vi "CRYGraph XY Window.vi"() -> ()   [LabVIEW 2013]
uses:
  <vilib>/Utility/miscctls.llb/LVPoint32TypeDef.ctl
  Control/CRYFlag Cluster.ctl
  <vilib>/Utility/miscctls.llb/LVRowAndColumnTypeDef.ctl
  <vilib>/Utility/miscctls.llb/LVRectTypeDef.ctl
  CRYCurveLibrary/Global/CRYCurve Library Global.vi
  SubVI/CRYData View Global.vi
  SubVI/CRYMain Sub Window Global.vi
panel:
  in  "GraphClick":bool
  out "AxisChangeOption":string
  out "PhaseShow":bool=TRUE
  in  "WhichKey":string
  out "KeyRepeatCount":i32
  in  "CursorMoveFinish":bool
  out "LegendVScrollShow":bool=TRUE
  out "Legend Ref":refnum<vi>
  out "SelectedRow":i32[](array[numeric])
  in  "LoadFinish":bool
  in  "ScaleFitY 2":bool
  in  "ScaleFitY":bool
  in  "ScaleFitX":bool
  in  "ToolbarUpdate":bool
  in  "OpenProperty":bool
  out "PropertyTab":string
  in  "PaletteShow":bool
  out "PreviewScaleMin":dbl
  out "PreviewScaleMax":dbl
  in  "FitPanes":bool
  in  "DirectionKey":bool
  out "MagnitudeShow":bool=TRUE
  out "Graph Ref":refnum<vi>
  out "PreviewGraph Ref":refnum<vi>
  out "PreviewCoords":T1
  in  "ScaleRange":bool
  out "Repaint Watermark":i32
  out "Event Name":string
  out "ReportDrop":bool
  in  "AxisChange":bool
  in  "RemoveSome":bool
  out "ScaleMin":dbl
  out "ScaleMax":dbl
  out "ScrollTick Ref":refnum<vi>
  out "Scrollbar Ref":refnum<vi>
  in  "PreviewShow":bool
  in  "RemoveAll":bool
  in  "CursorColor":bool
  out "NewCursIdx":u32
  out "Test":string
  in  "OldCursIdx":u32
  out "Queue Name":string
  in  "StateOut":bool
  out "Cursor Coords":T1
  in  "CursorPlot":bool
  out "Cursor Ref":refnum<vi>
  in  "CursorShow":bool
  out "XY Graph":cluster{"XY Graph":cluster{dbl, dbl}[]}[](graph)
  out "Title Name":string
  out "OldRow":i32
  out "TotalPlot":u32
  out "Graph Number":i32
  in  "stop":bool
  out "PreviewGraph":cluster{"XY Graph":cluster{dbl, dbl}[]}[](graph)
  in  "CursorEnabled":bool
  in  "Scrollbar":dbl(c297)
  in  "ScrollTick":dbl(slide) scale=0.0..1.0 scale format="%-#3.2p"
  in  "Cursor":string[][](table)
  in  "LegendShow":bool
  in  "ColorBox":u32(colorbox)
  in  "Legend":i32[](listbox)
  in  "GraphType":string
types:
  T1 = typedef "LVPoint32TypeDef.ctl" = cluster{"Horizontal":i32, "Vertical":i32}
  T2 = typedef "CRYFlag Cluster.ctl" = cluster{"LegendShow":bool, "CellClick":bool, "Total Number":bool, "ScaleFitX":bool, "ScaleFitY":bool, "MapModeX":u8, "MapModeY":u8, "CursorShow":bool, "MagnitudeShow":bool, "PreviewShow":bool, "CursorEnabled":bool, "IntensityShow":bool, "PaletteShow":bool, "PhaseShow":bool, "XYShow":bool, "FrequencyShow":bool, "LegendVScrollShow":bool, "FrequencyVScrollShow":bool}
  T3 = typedef "CRYGraph Event.ctl" = cluster{"EvenName":string, "TitleName":string, "GraphName":string, "GraphType":string, "Data":variant, "Queue Name":string, "DataView Number":i32}
  T4 = enum16{"No Scaling", "Scale All Objects", "Scale Single Object"}
  T5 = typedef "LVRowAndColumnTypeDef.ctl" = cluster{"Row":i32, "Column":i32}
  T6 = typedef "LVRectTypeDef.ctl" = cluster{"Left":i16, "Top":i16, "Right":i16, "Bottom":i16}
  T7 = typedef "LVBoundsTypeDef.ctl" = cluster{"Width":u32, "Height":u32}
  T8 = typedef "LVPositionTypeDef.ctl" = cluster{"Left":i32, "Top":i32}
  T9 = typedef "CRYData Cluster.ctl" = cluster{"Name":string, "Curve":cluster{"x":dbl, "y":dbl, "z":dbl}[], "X data":u16, "Y data":u16, "Z data":u16, "X axis":u16, "Y axis":u16, "Z axis":u16, "X unit":string, "Y unit":string, "Z unit":string, "X dB ref":dbl, "Y dB ref":dbl, "Z dB ref":dbl, "single val":bool, "protected":bool, "display X":bool, "display Y":bool, "display Z":bool, "Test Info":string, "Step No.":i32, "Plot Settings":cluster{"Color":u32, "Interpolation":u8, "Point Style":u8, "Line Style":u8, "Point Color":u32, "Line Width":u8, "Bar Plot Style":u8, "Fill To":i16}, "AutoProtect":bool}
  T10 = typedef "LVRangeTypeDef.ctl" = cluster{"Minimum":dbl, "Maximum":dbl, "Increment":dbl, "Minor Increment":dbl, "Start":dbl}
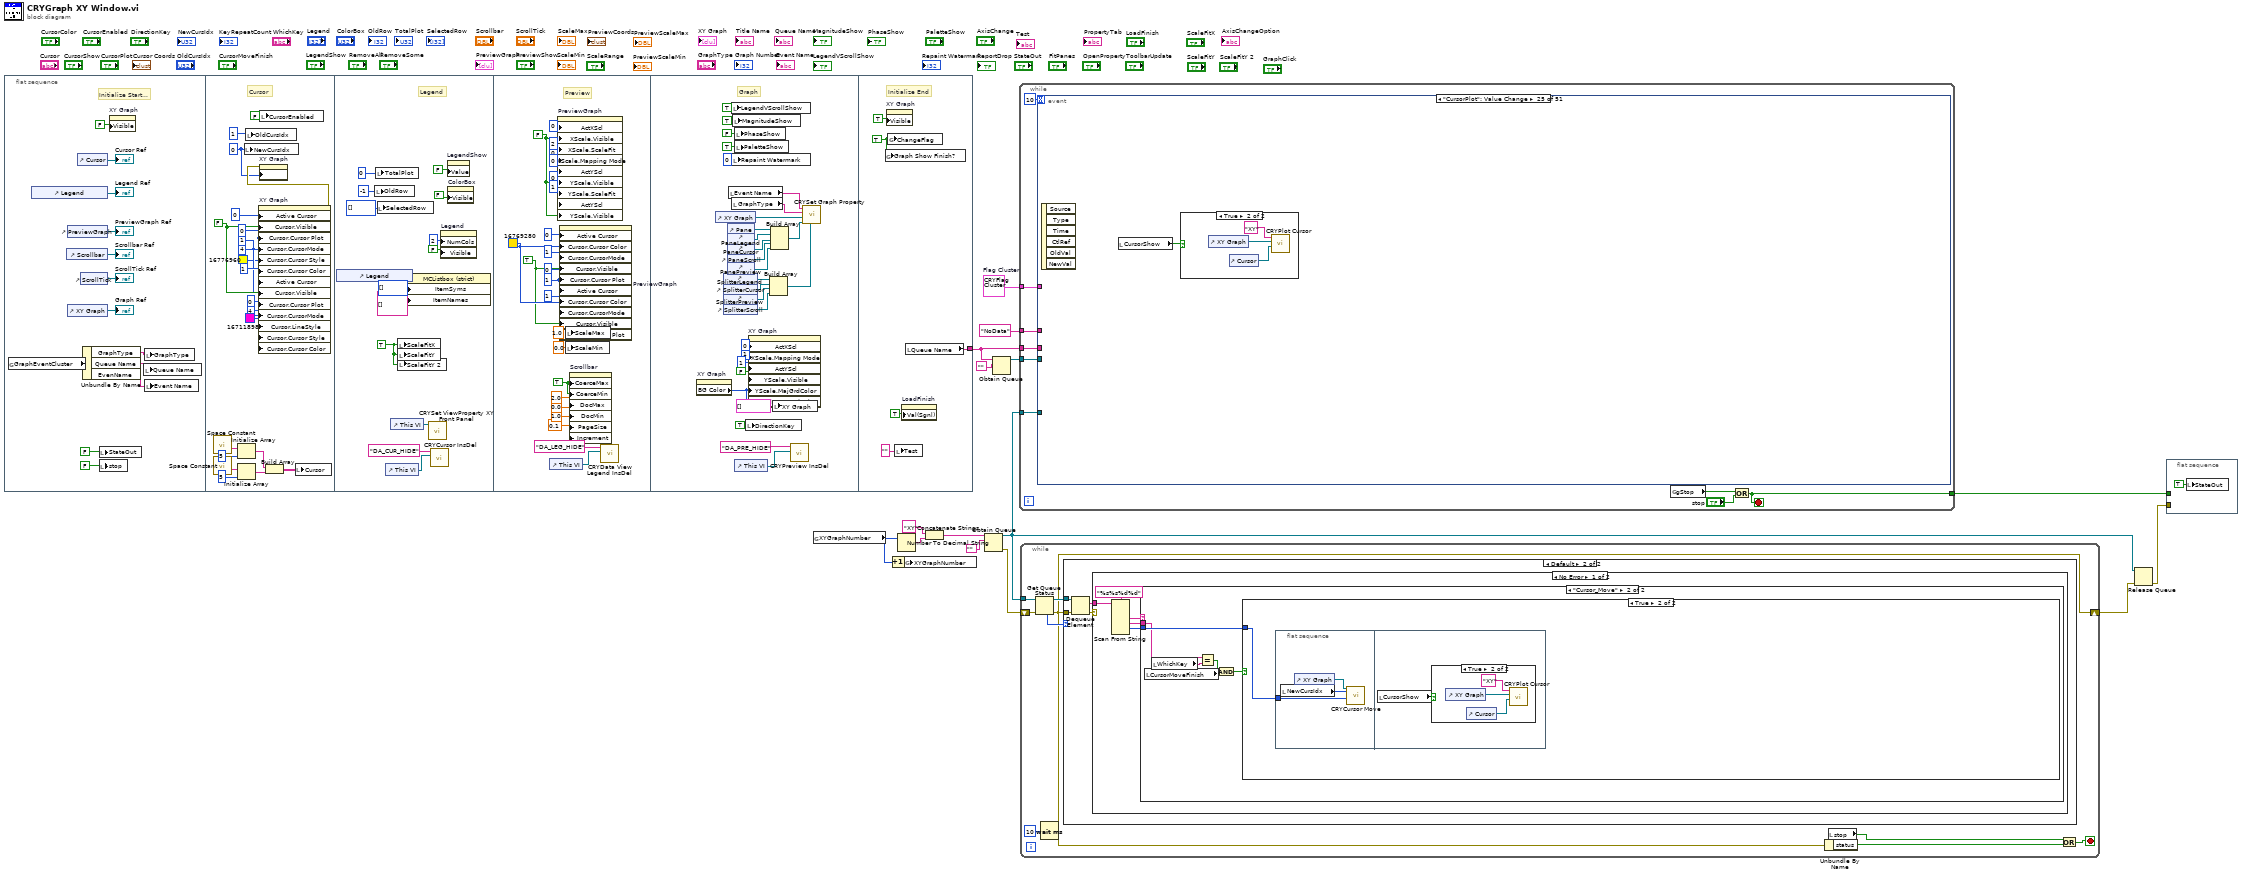
[diagram p0: block diagram]
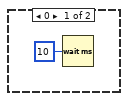
[diagram p2: hidden frame]
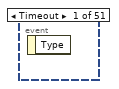
[diagram p7: hidden frame]
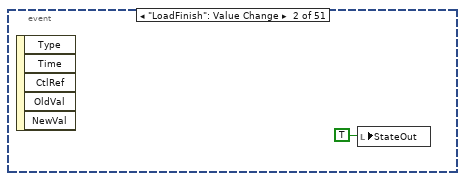
[diagram p8: hidden frame]
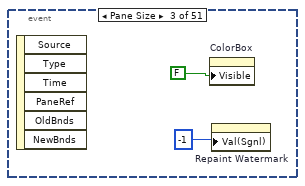
[diagram p9: hidden frame]
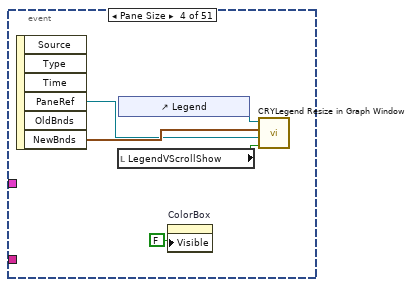
[diagram p10: hidden frame]
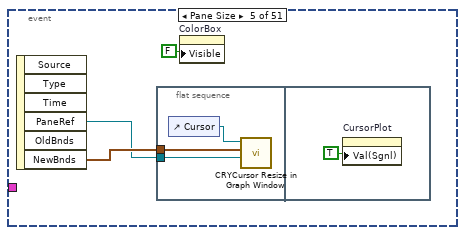
[diagram p11: hidden frame]
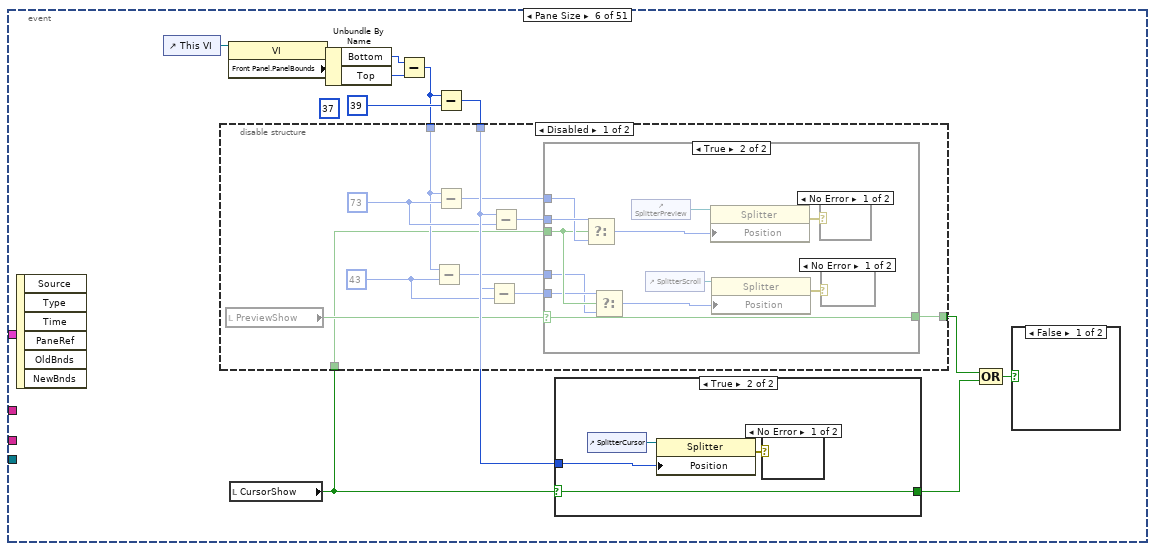
[diagram p12: hidden frame]
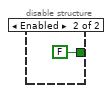
[diagram p16: hidden frame]
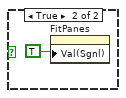
[diagram p17: hidden frame]
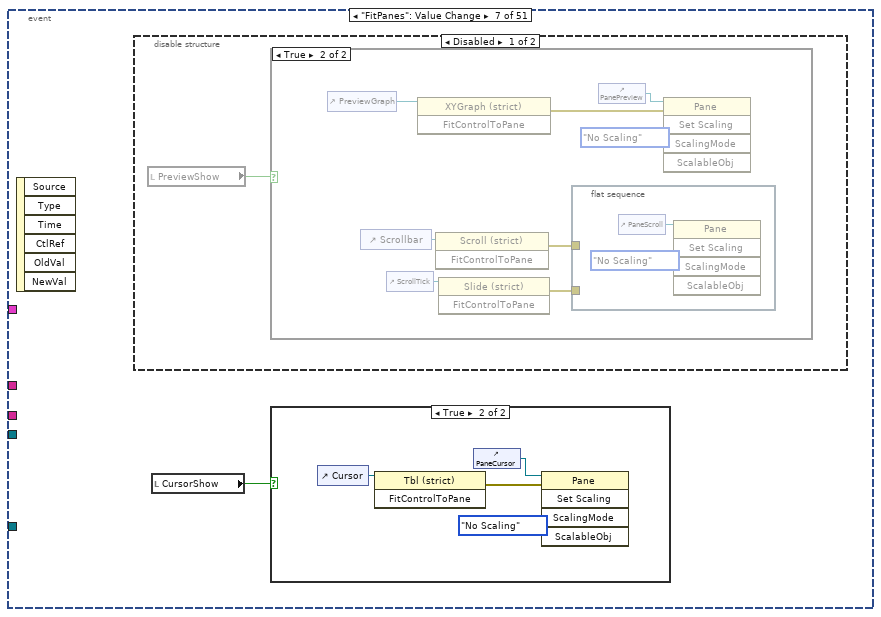
[diagram p20: hidden frame]
diagram:
  w14 = T2 {"LegendShow"=FALSE, "CellClick"=FALSE, "Total Number"=FALSE, "ScaleFitX"=FALSE, "ScaleFitY"=FALSE, "MapModeX"=0, "MapModeY"=0, "CursorShow"=FALSE, "MagnitudeShow"=FALSE, "PreviewShow"=FALSE, "CursorEnabled"=FALSE, "IntensityShow"=FALSE, "PaletteShow"=FALSE, "PhaseShow"=FALSE, "XYShow"=FALSE, "FrequencyShow"=FALSE, "LegendVScrollShow"=FALSE, "FrequencyVScrollShow"=FALSE}  # Flag Cluster
  n1 = flat-sequence {
    tunnel: [w117] -> w12
    frame #0 {
      # "Initialize Start..."
      n2 = global read "CRYData View Global.vi" "GraphEventCluster"() -> (w23:T3)
      n3 = control-ref of="Legend"() -> (→"Legend Ref":refnum<vi>)
      n4 = control-ref of="Scrollbar"() -> (→"Scrollbar Ref":refnum<vi>)
      n5 = control-ref of="PreviewGraph"() -> (→"PreviewGraph Ref":refnum<vi>)
      n6 = control-ref of="XY Graph"() -> (→"Graph Ref":refnum<vi>)
      n7 = control-ref of="Cursor"() -> (→"Cursor Ref":refnum<vi>)
      n8 = control-ref of="ScrollTick"() -> (→"ScrollTick Ref":refnum<vi>)
      n9 = Unbundle By Name(w23) -> ("GraphType"=w21:string, "Queue Name"=w22:string, "EvenName"=w20:string)
      n10 = local write "StateOut"(FALSE ("StateOut")) -> ()
      n11 = local write "stop"(FALSE ("stop")) -> ()
      n12 = property on="XY Graph" class="XYGraph (strict)"("Visible"=FALSE) -> ()  [unwired: 2 in, 2 out]
      n13 = local write "Queue Name"(w22) -> ()
      n14 = local write "GraphType"(w21) -> ()
      n15 = local write "Event Name"(w20) -> ()
    }
    frame #1 {
      w34 = u32 0 ("Active Cursor")
      w36 = u32 1 ("Cursor.Cursor Mode")
      w37 = 0 ("Cursor.Cursor Plot")
      w38 = FALSE ("Cursor.Visible")
      # "Cursor"
      n16 = call <vilib>:"Space Constant.vi"() -> ("String"=w44:string)
      n17 = call <vilib>:"Space Constant.vi"() -> ("String"=w49:string)
      n18 = Initialize Array(w44, 5 ("dimension size")) -> (w46:string[])
      n19 = Initialize Array(w49, 5 ("dimension size")) -> (w50:string[])
      n20 = local write "NewCursIdx"(w34) -> ()
      n21 = local write "OldCursIdx"(u32 1 ("OldCursIdx")) -> ()
      n22 = property on="XY Graph" class="XYGraph (strict)"("Active Cursor"=u32 0, "Cursor.Visible"=w38, "Cursor.Cursor Plot"=w37, "Cursor.CursorMode"=w36, "Cursor.Cursor Style"=u8 4, "Cursor.Cursor Color"=u32 16776960, "Active Cursor"=u32 1, "Cursor.Visible"=w38, "Cursor.Cursor Plot"=w37, "Cursor.CursorMode"=w36, "Cursor.LineStyle"=u8 0 ("Cursor.Line Style"), "Cursor.Cursor Style"=u8 4, "Cursor.Cursor Color"=u32 16711898) -> (error out=w35:errorcluster)  [unwired: 2 in, 1 out]
      n23 = property on="XY Graph" class="XYGraph (strict)"(error in=w35, "Active Cursor"=w34) -> ()  [unwired: 1 in, 2 out]
      n24 = local write "CursorEnabled"(FALSE ("CursorEnabled")) -> ()
      n25 = Build Array(w46, w50) -> (w47:string[][])
      n26 = local write "Cursor"(w47) -> ()
    }
    frame #2 {
      w52 = TRUE ("ScaleFitX")
      # "Legend"
      n27 = control-ref of="Legend"() -> (w64:refnum<vi>)
      n28 = local write "OldRow"(-1 ("OldRow 2")) -> ()
      n29 = local write "TotalPlot"(u32 0 ("TotalPlot")) -> ()
      n30 = local write "SelectedRow"(i32[] [] ("SelectedRow")) -> ()
      n31 = control-ref of="This VI"() -> (w55:refnum<vi>)
      n32 = control-ref of="This VI"() -> (w53:refnum<vi>)
      n33 = local write "ScaleFitX"(w52) -> ()
      n34 = local write "ScaleFitY"(w52) -> ()
      n35 = local write "ScaleFitY 2"(w52) -> ()
      n36 = property on="Property Node" class="MCListbox (strict)"(reference=w64, "ItemSyms"=i32[] [] ("Item Symbols"), "ItemNames"=string[][] [] ("Item Names")) -> ()  [unwired: 1 in, 2 out]
      n37 = call "CRYSet ViewProperty XY  Front Panel.vi"("Vi Ref"=w53) -> ()  [unwired: 11 in]
      n38 = call "CRYCursor InsDel.vi"("Graph VI Ref"=w55, "sAction"="DA_CUR_HIDE" ("Action Type")) -> ()  [unwired: 10 in]
      n39 = property on="Legend" class="MCListbox (strict)"("NumCols"=u32 2 ("Number of Columns"), "Visible"=FALSE) -> ()  [unwired: 2 in, 2 out]
      n40 = property on="LegendShow" class="Bool (strict)"("Value"=FALSE ("Visible")) -> ()  [unwired: 2 in, 2 out]
      n41 = property on="ColorBox" class="ColBox"("Visible"=FALSE) -> ()  [unwired: 2 in, 2 out]
    }
    frame #3 {
      w72 = 0 ("Cursor.Cursor Plot")
      w68 = u32 16769280
      w67 = TRUE ("Cursor.Visible")
      w65 = FALSE ("X Scale.Visible")
      w87 = TRUE ("Coerce Maximum Value")
      # "Preview"
      n42 = control-ref of="This VI"() -> (w75:refnum<vi>)
      n43 = property on="PreviewGraph" class="XYGraph (strict)"("ActXScl"=0 ("Active X Scale"), "XScale.Visible"=w65, "XScale.ScaleFit"=u8 2 ("X Scale.Scale Fit"), "XScale.Mapping Mode"=u8 0 ("X Scale.Mapping Mode"), "ActYScl"=0 ("Active Y Scale"), "YScale.Visible"=w65, "YScale.ScaleFit"=u8 0 ("Y Scale.Scale Fit"), "ActYScl"=1 ("Active Y Scale"), "YScale.Visible"=w65) -> ()  [unwired: 2 in, 2 out]
      n44 = property on="PreviewGraph" class="XYGraph (strict)"("Active Cursor"=u32 0, "Cursor.Cursor Color"=w68, "Cursor.CursorMode"=u32 1 ("Cursor.Cursor Mode"), "Cursor.Visible"=w67, "Cursor.Cursor Plot"=w72, "Active Cursor"=u32 1, "Cursor.Cursor Color"=w68, "Cursor.CursorMode"=u32 1 ("Cursor.Cursor Mode"), "Cursor.Visible"=w67, "Cursor.Cursor Plot"=w72) -> ()  [unwired: 2 in, 2 out]
      n45 = local write "ScaleMax"(1.0 ("ScaleMax")) -> ()
      n46 = local write "ScaleMin"(0.0 ("ScaleMin")) -> ()
      n47 = property on="Scrollbar" class="Scroll (strict)"("CoerceMax"=w87, "CoerceMin"=w87, "DocMax"=2.0 ("Doc Max"), "DocMin"=0.0 ("Doc Min"), "PageSize"=1.0 ("Page Size"), "Increment"=0.1) -> ()  [unwired: 2 in, 2 out]
      n48 = call "CRYData View Legend InsDel.vi"("Graph VI Ref"=w75, "sAction"="DA_LEG_HIDE" ("Action Type")) -> ()  [unwired: 2 in, 8 out]
    }
    frame #4 {
      # "Graph"
      n49 = property on="XY Graph" class="XYGraph (strict)"() -> ("BG Color"=w113:u32)  [unwired: 2 in, 2 out]
      n50 = control-ref of="XY Graph"() -> (w96:refnum<vi>)
      n51 = control-ref of="SplitterLegend"() -> (w110:refnum<vi>)
      n52 = control-ref of="SplitterCursor"() -> (w109:refnum<vi>)
      n53 = control-ref of="SplitterPreview"() -> (w108:refnum<vi>)
      n54 = control-ref of="SplitterScroll"() -> (w107:refnum<vi>)
      n55 = control-ref of="Pane"() -> (w106:refnum<vi>)
      n56 = control-ref of="PaneLegend"() -> (w102:refnum<vi>)
      n57 = control-ref of="PaneCursor"() -> (w105:refnum<vi>)
      n58 = control-ref of="PaneScroll"() -> (w104:refnum<vi>)
      n59 = control-ref of="PanePreview"() -> (w103:refnum<vi>)
      n60 = local read "Event Name"() -> (w98:string)
      n61 = local write "LegendVScrollShow"(TRUE ("LegendVScrollShow")) -> ()
      n62 = local write "Repaint Watermark"(0 ("Repaint Watermark")) -> ()
      n63 = local read "GraphType"() -> (w99:string)
      n64 = local write "MagnitudeShow"(TRUE ("Magnitude")) -> ()
      n65 = local write "PhaseShow"(FALSE ("PhaseShow")) -> ()
      n66 = local write "PaletteShow"(TRUE ("PaletteShow")) -> ()
      n67 = control-ref of="This VI"() -> (w111:refnum<vi>)
      n68 = local write "DirectionKey"(TRUE ("DirectionKey")) -> ()
      n69 = property on="XY Graph" class="XYGraph (strict)"("ActXScl"=0 ("Active X Scale"), "XScale.Mapping Mode"=u8 1 ("X Scale.Mapping Mode"), "ActYScl"=1 ("Active Y Scale"), "YScale.Visible"=FALSE ("Y Scale.Visible"), "YScale.MajGrdColor"=w113, "YScale.MnrGrdColor"=w113) -> ()  [unwired: 2 in, 2 out]
      n70 = Build Array(w110, w109, w108, w107) -> (w100:refnum<vi>[])
      n71 = Build Array(w106, w102, w105, w104, w103) -> (w101:refnum<vi>[])
      n72 = local write "XY Graph"(cluster{"XY Graph":cluster{dbl, dbl}[]}[] [] ("XY Graph")) -> ()
      n73 = call "CRYPreview InsDel.vi"("Graph VI Ref"=w111, "sAction"="DA_PRE_HIDE" ("Action Type")) -> ()  [unwired: 10 in]
      n74 = call "CRYSet Graph Property.vi"("Splitters"=w100, "Panes"=w101, "Graph Ref"=w96, "Graph Type"=w99, "Event Name"=w98) -> ()  [unwired: 7 in]
    }
    frame #5 {
      w120 = TRUE ("ChangeFlag")
      # "Initialize End"
      n75 = global write "CRYData View Global.vi" "Graph Show Finish?"(w120) -> ()
      n76 = property on="XY Graph" class="XYGraph (strict)"("Visible"=TRUE) -> ()  [unwired: 2 in, 2 out]
      n77 = global write "CRYData View Global.vi" "ChangeFlag"(w120) -> ()
      n78 = local write "Test"("" ("Test")) -> ()
      n79 = property on="LoadFinish" class="Bool (strict)"("Val(Sgnl)"=TRUE ("Value (Signaling)")) -> ()  [unwired: 2 in, 2 out]
      n80 = local read "Queue Name"() -> (w117:string)
    }
  }
  n81 = global read "CRYCurve Library Global.vi" "XYGraphNumber"() -> (w4:u32)
  n82 = Increment(x=w4) -> (x+1=w3:u32)
  n83 = Number To Decimal String(number=w4) -> (decimal integer string=w5:string)  [unwired: 1 in]
  n84 = global write "CRYCurve Library Global.vi" "XYGraphNumber"(w3) -> ()
  n85 = Concatenate Strings("XY" ("YAxisTitle"), w5) -> (w7:string)
  n86 = Obtain Queue(name (unnamed)=w7, element data type="" ("Action Type")) -> (queue out=w1:refnum<queue>, error out=w10:errorcluster)  [unwired: 3 in, 1 out]
  n87 = Obtain Queue(name (unnamed)=w12, element data type="") -> (queue out=w16:refnum<queue>)  [unwired: 3 in, 2 out]
  n88 = while {
    tunnel: w16 -> [w129]
    tunnel: w14 -> [w127]
    tunnel: "NoData" ("input 2") -> [w124]
    tunnel: w12 -> [w123]
    tunnel: [w122] -> w11
    tunnel: w1 -> [w121]
    stop <- w122 stop-if-true
    n89 = event shown="[24] \"CursorPlot\": Value Change" {
      selector: _ -> [_ _ _ _ _ _ _ _ _ _ _ _ _ _ _ _ _ _ _ _ _ _ _ _ _ _ _ _ _ _ _ _ _ _ _ _ _ _ _ _ _ _ _ _ _ _ _ _ _ _ _]
      dyn-events: _ -> [_ _ _ _ _ _ _ _ _ _ _ _ _ _ _ _ _ _ _ _ _ _ _ _ _ _ _ _ _ _ _ _ _ _ _ _ _ _ _ _ _ _ _ _ _ _ _ _ _ _ _]
      timeout: 10 -> [_ _ _ _ _ _ _ _ _ _ _ _ _ _ _ _ _ _ _ _ _ _ _ _ _ _ _ _ _ _ _ _ _ _ _ _ _ _ _ _ _ _ _ _ _ _ _ _ _ _ _]
      tunnel: w129 -> [_ _ _ _ _ _ _ w205 w210 _ w246 _ w454 _ w507 _ _ _ _ _ _ _ _ _ _ _ _ _ _ _ _ w810 _ _ _ _ _ w1065 _ _ w1078 _ _ _ _ _ _ _ _ _ _]
      tunnel: w127 -> [_ _ _ _ _ _ _ _ _ w230 _ w431 _ w492 _ w550 _ _ _ _ _ _ _ _ _ _ _ _ _ _ _ _ _ _ _ _ _ _ _ _ _ _ _ _ _ _ _ _ _ _ _]
      tunnel: w124 -> [_ _ _ _ _ _ _ _ _ _ w248 _ w451 _ w506 _ _ _ _ _ _ _ _ _ _ _ _ _ _ _ _ _ _ _ _ _ _ _ _ _ _ _ _ _ _ _ _ _ _ _ _]
      tunnel: w123 -> [_ _ _ _ _ _ _ _ _ w223 w247 _ _ _ _ _ _ _ _ _ _ _ _ _ _ _ _ _ _ _ _ _ _ _ _ _ _ _ _ _ _ _ _ _ _ _ _ _ _ _ _]
      tunnel: w121 -> [_ _ _ _ _ _ _ _ _ _ _ _ _ _ _ _ _ _ w634 w653 w668 _ _ _ _ _ _ _ _ _ _ _ _ _ _ _ _ _ _ _ _ _ _ _ _ _ _ _ _ _ _]
      event Timeout {
        n90 = event-data() -> ()  [unwired: 2 out]
      }
      event "LoadFinish": Value Change {
        n91 = event-data() -> ()  [unwired: 6 out]
        n92 = local write "StateOut"(TRUE ("StateOut")) -> ()
      }
      event Pane Size {
        n93 = event-data() -> ()  [unwired: 7 out]
        n94 = property on="ColorBox" class="ColBox"("Visible"=FALSE) -> ()  [unwired: 2 in, 2 out]
        n95 = property on="Repaint Watermark" class="DigNum (strict)"("Val(Sgnl)"=-1 ("y")) -> ()  [unwired: 2 in, 2 out]
      }
      event Pane Size {
        n96 = event-data() -> ("PaneRef"=w135:refnum<vi>, "NewBnds"=w136:T6)  [unwired: 5 out]
        n97 = local read "LegendVScrollShow"() -> (w133:bool)
        n98 = control-ref of="Legend"() -> (w134:refnum<vi>)
        n99 = property on="ColorBox" class="ColBox"("Visible"=FALSE) -> ()  [unwired: 2 in, 2 out]
        n100 = call "CRYLegend Resize in Graph Window.vi"("VScrollShow"=w133, "Pane Ref"=w135, "input cluster"=w136, "Legend"=w134) -> ()  [unwired: 8 out]
      }
      event Pane Size {
        n101 = event-data() -> ("PaneRef"=w139:refnum<vi>, "NewBnds"=w140:T6)  [unwired: 5 out]
        n102 = flat-sequence {
          tunnel: w140 -> [w143]
          tunnel: w139 -> [w141]
          frame #0 {
            n103 = control-ref of="Cursor"() -> (w142:refnum<vi>)
            n104 = call "CRYCursor Resize in Graph Window.vi"("Pane Ref"=w141, "input cluster"=w143, "Graph Cursor Ref"=w142) -> ()  [unwired: 9 in]
          }
          frame #1 {
            n105 = property on="CursorPlot" class="Bool (strict)"("Val(Sgnl)"=TRUE ("Value (Signaling)")) -> ()  [unwired: 2 in, 2 out]
          }
        }
        n106 = property on="ColorBox" class="ColBox"("Visible"=FALSE) -> ()  [unwired: 2 in, 2 out]
      }
      event Pane Size {
        (unwired) 37
        n107 = event-data() -> ()  [unwired: 7 out]
        n108 = control-ref of="This VI"() -> (w149:refnum<vi>)
        n109 = property class="VI"(reference=w149) -> ("Front Panel.PanelBounds"=w150:T6)  [unwired: 1 in, 2 out]
        n110 = local read "CursorShow"() -> (w146:bool)
        n111 = Unbundle By Name(w150) -> ("Bottom"=w147:i16, "Top"=w148:i16)
        n112 = Subtract(x=w147, y=w148) -> (x-y=w151:i16)
        n113 = Subtract(x=w151, y=39) -> (x-y=w155:i32)
        n114 = disable-structure shown="Disabled" {
          disable-tunnel: w155 -> [w163 _]
          disable-tunnel: [w161 FALSE] -> w152
          disable-tunnel: w151 -> [w158 _]
          disable-tunnel: w146 -> [w156 _]
          frame Disabled {
            w164 = 43
            w162 = 73
            n115 = local read "PreviewShow"() -> (w157:bool)
            n116 = Subtract(x=w158, y=w164) -> (x-y=w160:i32)
            n117 = Subtract(x=w158, y=w162) -> (x-y=w159:i32)
            n118 = Subtract(x=w163, y=w164) -> (x-y=w166:i32)
            n119 = Subtract(x=w163, y=w162) -> (x-y=w165:i32)
            n120 = case shown="True" w157 {
              selector: w157 -> [w167 w177]
              tunnel: w159 -> [_ w175]
              tunnel: w160 -> [_ w171]
              tunnel: [w167 w177] -> w161
              tunnel: w156 -> [_ w173]
              tunnel: w165 -> [_ w176]
              tunnel: w166 -> [_ w172]
              frame False {
              }
              frame True {
                n121 = Select(t=w176, s=w173, f=w175) -> (s? t:f=w174:i32)
                n122 = Select(t=w172, s=w173, f=w171) -> (s? t:f=w170:i32)
                n123 = control-ref of="SplitterPreview"() -> (w169:refnum<vi>)
                n124 = control-ref of="SplitterScroll"() -> (w168:refnum<vi>)
                n125 = property class="Splitter"(reference=w169, "Position"=w174) -> (error out=w179:errorcluster)  [unwired: 1 in, 1 out]
                n126 = property class="Splitter"(reference=w168, "Position"=w170) -> (error out=w178:errorcluster)  [unwired: 1 in, 1 out]
                n127 = case shown="No Error" w179 {
                  frame No Error {
                  }
                  frame Error {
                  }
                }
                n128 = case shown="No Error" w178 {
                  frame No Error {
                  }
                  frame Error {
                  }
                }
              }
            }
          }
          frame Enabled {
          }
        }
        n129 = case shown="True" w146 {
          selector: w146 -> [w182 w184]
          tunnel: w155 -> [_ w186]
          tunnel: [w182 w184] -> w153
          frame False {
          }
          frame True {
            n130 = control-ref of="SplitterCursor"() -> (w183:refnum<vi>)
            n131 = property class="Splitter"(reference=w183, "Position"=w186) -> (error out=w185:errorcluster)  [unwired: 1 in, 1 out]
            n132 = case shown="No Error" w185 {
              frame No Error {
              }
              frame Error {
              }
            }
          }
        }
        n133 = Compound Arithmetic op=OR(w152, w153) -> (w145:bool)
        n134 = case shown="False" w145 {
          frame False {
          }
          frame True {
            n135 = property on="FitPanes" class="Bool (strict)"("Val(Sgnl)"=TRUE ("Value (Signaling)")) -> ()  [unwired: 2 in, 2 out]
          }
        }
      }
      event "FitPanes": Value Change {
        n136 = event-data() -> ()  [unwired: 7 out]
        n137 = disable-structure shown="Disabled" {
          frame Disabled {
            n138 = local read "PreviewShow"() -> (w188:bool)
            n139 = case shown="True" w188 {
              frame False {
              }
              frame True {
                n140 = control-ref of="PreviewGraph"() -> (w195:refnum<vi>)
                n141 = control-ref of="Scrollbar"() -> (w194:refnum<vi>)
                n142 = control-ref of="ScrollTick"() -> (w193:refnum<vi>)
                n143 = invoke class="XYGraph (strict)" method="FitControlToPane"(reference=w195) -> (error out=w192:errorcluster)  [unwired: 2 in, 2 out]
                n144 = invoke class="Scroll (strict)" method="FitControlToPane"(reference=w194) -> (error out=w191:errorcluster)  [unwired: 2 in, 2 out]
                n145 = invoke class="Slide (strict)" method="FitControlToPane"(reference=w193) -> (error out=w190:errorcluster)  [unwired: 2 in, 2 out]
                n146 = flat-sequence {
                  tunnel: w191 -> [_]
                  tunnel: w190 -> [_]
                  frame #0 {
                    n147 = control-ref of="PaneScroll"() -> (w197:refnum<vi>)
                    n148 = invoke class="Pane" method="Set Scaling"(reference=w197, "ScalingMode"=T4."No Scaling" ("Scaling Mode")) -> ()  [unwired: 3 in, 5 out]
                  }
                }
                n149 = control-ref of="PanePreview"() -> (w189:refnum<vi>)
                n150 = invoke class="Pane" method="Set Scaling"(reference=w189, error in=w192, "ScalingMode"=T4."No Scaling" ("Scaling Mode")) -> ()  [unwired: 2 in, 5 out]
              }
            }
          }
          frame Enabled {
          }
        }
        n151 = local read "CursorShow"() -> (w187:bool)
        n152 = case shown="True" w187 {
          frame False {
          }
          frame True {
            n153 = control-ref of="Cursor"() -> (w202:refnum<vi>)
            n154 = invoke class="Tbl (strict)" method="FitControlToPane"(reference=w202) -> (error out=w201:errorcluster)  [unwired: 2 in, 2 out]
            n155 = control-ref of="PaneCursor"() -> (w199:refnum<vi>)
            n156 = invoke class="Pane" method="Set Scaling"(reference=w199, error in=w201, "ScalingMode"=T4."No Scaling" ("Scaling Mode")) -> ()  [unwired: 2 in, 5 out]
          }
        }
      }
      event Mouse Down {
        n157 = event-data() -> ()  [unwired: 8 out]
        n158 = local read "Test"() -> (w204:string)
        n159 = global write "CRYCurve Library Global.vi" "Graph Inner Click"(TRUE ("Graph Inner Click")) -> ()
        n160 = case shown="Default" w204 {
          tunnel: w205 -> [w208 _]
          frame Default {
            n161 = control-ref of="This VI"() -> (w206:refnum<vi>)
            n162 = call "CRYMouse Down in Graph Window.vi"("Queue"=w208, "Selected Type"=enum16{"Curves", "Values", "Results", "WFM"}."Curves" ("Type"), "pGraph VI In"=w206) -> ()  [unwired: 3 in, 6 out]
          }
          frame "Test" {
          }
        }
      }
      event "GraphClick": Value Change {
        n163 = event-data() -> ()  [unwired: 7 out]
        n164 = global read "CRYCurve Library Global.vi" "Graph Inner Click"() -> (w209:bool)
        n165 = case shown="True" w209 {
          tunnel: w210 -> [w213 _]
          frame False {
            n166 = control-ref of="This VI"() -> (w211:refnum<vi>)
            n167 = call "CRYMouse Down in Graph Window.vi"("Queue"=w213, "Selected Type"=enum16{"Curves", "Values", "Results", "WFM"}."Curves" ("Type"), "pGraph VI In"=w211) -> ()  [unwired: 3 in, 6 out]
          }
          frame True {
            n168 = global write "CRYCurve Library Global.vi" "Graph Inner Click"(FALSE ("Graph Inner Click")) -> ()
          }
        }
      }
      event Shortcut Menu Activation? {
        n169 = event-data() -> ("MenuRef"=w232:refnum<k9>)  [unwired: 1 out]
        n170 = local read "MagnitudeShow"() -> (w219:bool)
        n171 = local read "CursorEnabled"() -> (w225:bool)
        n172 = property on="XY Graph" class="XYGraph (strict)"() -> ("XScale.Mapping Mode"=w228:u8, "YScale.Mapping Mode"=w227:u8)  [unwired: 2 in, 2 out]
        n173 = local read "PreviewShow"() -> (w224:bool)
        n174 = local read "LegendShow"() -> (w231:bool)
        n175 = local read "PaletteShow"() -> (w218:bool)
        n176 = local read "CursorShow"() -> (w226:bool)
        n177 = local read "PhaseShow"() -> (w215:bool)
        n178 = local read "ScaleFitX"() -> (w217:bool)
        n179 = local read "ScaleFitY"() -> (w216:bool)
        n180 = Bundle By Name(cluster=w230, "LegendShow"=w231, "ScaleFitX"=w217, "ScaleFitY"=w216, "MapModeX"=w228, "MapModeY"=w227, "CursorShow"=w226, "PreviewShow"=w224, "CursorEnabled"=w225, "MagnitudeShow"=w219, "PaletteShow"=w218, "PhaseShow"=w215) -> (w229:T2)
        n181 = local read "Test"() -> (w220:string)
        n182 = case shown="Default" w220 {
          tunnel: w223 -> [_ w238]
          tunnel: ["" ("sData Out") w237] -> w222
          tunnel: [TRUE ("bResult Out") w236] -> w221
          frame "Test" {
          }
          frame Default {
            n183 = local read "Graph Number"() -> (w235:i32)
            n184 = call "CRYGraph View Socket Client.vi"("sOption"="MENUOPTION", "nData"=w235, "sData"=w238, "sAction"="GET_GRAPHDATA") -> ("bResult Out"=w236:bool, "sData Out"=w237:string)  [unwired: 4 in, 2 out]
          }
        }
        n185 = case shown="True" w221 {
          tunnel: w232 -> [_ w245]
          tunnel: w229 -> [_ w243]
          tunnel: w222 -> [_ w242]
          frame False {
          }
          frame True {
            n186 = control-ref of="This VI"() -> (w241:refnum<vi>)
            n187 = call "CRYGraph Window Menu.vi"("MenuOption"=w242, "pGraph VI"=w241, "Flag Cluster"=w243, "Type"="XY", "Runtime Menu Ref In"=w245) -> ()  [unwired: 7 out]
          }
        }
        n188 = event-data() -> ()  [unwired: 1 in, 2 out]
      }
      event Shortcut Menu Selection (User) {
        n189 = event-data() -> ("ItemTag"=w249:string)  [unwired: 1 out]
        n190 = case shown="\"DA_AXIS_MAG_HIDE\", \"DA_AXIS_MAG_VIEW\"" w249 {
          selector: w249 -> [w251 _ w337 w365 w397 w422 w427 _]
          tunnel: w248 -> [_ _ _ _ w391 _ _ _]
          tunnel: w247 -> [_ _ _ _ _ _ _ _]
          tunnel: w246 -> [_ _ _ _ w389 _ _ _]
          frame "DA_SCALE_X_A", "DA_SCALE_X_L", "DA_SCALE_Y_A", "DA_SCALE_Y_L" {
            n191 = case shown="\"DA_SCALE_X_A\", Default" w251 {
              selector: w251 -> [w255 w304 w308 w329]
              tunnel: [w255 w304 w308 w329] -> w250
              frame "DA_SCALE_X_A", Default {
                n192 = local read "ScaleFitX"() -> (w254:bool)
                n193 = Not(x=w254) -> (.not. x?=w253:bool)
                n194 = Select(t=u8 2, s=w253, f=u8 0) -> (s? t:f=w256:u8)
                n195 = property on="XY Graph" class="XYGraph (strict)"("XScale.ScaleFit"=w256) -> (error out=w257:errorcluster)  [unwired: 2 in, 1 out]
                n196 = disable-structure shown="Disabled" {
                  disable-tunnel: w257 -> [w261 _]
                  disable-tunnel: w256 -> [w260 _]
                  frame Disabled {
                    n197 = property on="PreviewGraph" class="XYGraph (strict)"("XScale.ScaleFit"=w260) -> ()  [unwired: 2 in, 2 out]
                    n198 = case shown="2" w260 {
                      tunnel: w261 -> [_ _]
                      frame Default {
                      }
                      frame 2 {
                        n199 = property on="XY Graph" class="XYGraph (strict)"() -> ("XScale.Maximum"=w290:dbl, "XScale.Minimum"=w291:dbl)  [unwired: 2 in, 2 out]
                        n200 = property on="PreviewGraph" class="XYGraph (strict)"() -> ("XScale.Maximum"=w271:dbl, "XScale.Minimum"=w265:dbl)  [unwired: 2 in, 2 out]
                        n201 = Greater?(x=w265, y=w291) -> (0:w292:bool)
                        n202 = Less?(x=w271, y=w290) -> (x < y?=w289:bool)
                        n203 = Subtract(x=w271, y=w265) -> (x-y=w270:dbl)
                        n204 = Select(t=w271, s=w289, f=w290) -> (s? t:f=w266:dbl)
                        n205 = Select(t=w265, s=w292, f=w291) -> (s? t:f=w267:dbl)
                        n206 = Subtract(x=w267, y=w265) -> (x-y=w264:dbl)
                        n207 = Subtract(x=w266, y=w265) -> (x-y=w263:dbl)
                        n208 = property on="PreviewGraph" class="XYGraph (strict)"("Active Cursor"=u32 0, "Cursor.Cursor X"=w267, "Active Cursor"=u32 1, "Cursor.Cursor X"=w266) -> (error out=w288:errorcluster)  [unwired: 2 in, 1 out]
                        n209 = Divide(x=w264, y=w270) -> (x/y=w268:dbl)
                        n210 = Divide(x=w263, y=w270) -> (x/y=w269:dbl)
                        n211 = property on="Scrollbar" class="Scroll (strict)"() -> ("DocMax"=w277:dbl, "PageSize"=w283:dbl)  [unwired: 2 in, 2 out]
                        n212 = Subtract(x=w268, y=w269) -> (x-y=w275:dbl)
                        n213 = flat-sequence {
                          tunnel: w288 -> [_]
                          frame #0 {
                            n214 = control-ref of="This VI"() -> (w294:refnum<vi>)
                            n215 = call "CRYPlot XY Graph Preview.vi"("sOption"="Move", "Graph VI Ref"=w294) -> ()  [unwired: 10 in]
                          }
                        }
                        n216 = Divide(x=w283, y=w275) -> (x/y=w274:dbl)
                        n217 = local read "ScaleMax"() -> (w273:dbl)
                        n218 = local read "ScaleMin"() -> (w272:dbl)
                        n219 = Add(x=w277, y=w274) -> (x+y=w276:dbl)
                        n220 = property on="Scrollbar" class="Scroll (strict)"("DocMin"=w276) -> ("DocMax"=w285:dbl, "DocMin"=w284:dbl)  [unwired: 2 in, 2 out]
                        n221 = Subtract(x=w273, y=w272) -> (x-y=w262:dbl)
                        n222 = Subtract(x=w268, y=w272) -> (x-y=w278:dbl)
                        n223 = Subtract(x=w285, y=w284) -> (x-y=w279:dbl)
                        n224 = Multiply(x=w278, y=w279) -> (x*y=w280:dbl)
                        n225 = Divide(x=w280, y=w262) -> (x/y=w281:dbl)
                        n226 = Add(x=w281, y=w284) -> (x+y=w282:dbl)
                        n227 = property on="Scrollbar" class="Scroll (strict)"("Value"=w282) -> ()  [unwired: 2 in, 2 out]
                      }
                    }
                  }
                  frame Enabled {
                  }
                }
                n228 = local write "ScaleFitX"(w253) -> ()
              }
              frame "DA_SCALE_Y_A" {
                n229 = local read "ScaleFitY"() -> (w296:bool)
                n230 = local read "ScaleFitY 2"() -> (w298:bool)
                n231 = Not(x=w296) -> (.not. x?=w295:bool)
                n232 = Not(x=w298) -> (.not. x?=w297:bool)
                n233 = Select(t=u8 2, s=w297, f=u8 0) -> (s? t:f=w301:u8)
                n234 = Select(t=u8 2, s=w295, f=u8 0) -> (s? t:f=w305:u8)
                n235 = local write "ScaleFitY"(w295) -> ()
                n236 = property on="XY Graph" class="XYGraph (strict)"("ActYScl"=1 ("Active Y Scale"), "YScale.ScaleFit"=w301) -> ()  [unwired: 2 in, 2 out]
                n237 = property on="XY Graph" class="XYGraph (strict)"("ActYScl"=0 ("Active Y Scale"), "YScale.ScaleFit"=w305) -> ()  [unwired: 2 in, 2 out]
                n238 = local write "ScaleFitY 2"(w297) -> ()
              }
              frame "DA_SCALE_X_L" {
                n239 = property on="XY Graph" class="XYGraph (strict)"() -> ("XScale.Mapping Mode"=w309:u8)  [unwired: 2 in, 2 out]
                n240 = Equal?(x=w309, y=u8 0) -> (x = y?=w314:bool)
                n241 = Select(t=u8 1, s=w314, f=u8 0) -> (s? t:f=w310:u8)
                n242 = property on="XY Graph" class="XYGraph (strict)"("XScale.Mapping Mode"=w310) -> ()  [unwired: 2 in, 2 out]
              }
              frame "DA_SCALE_Y_L" {
                n243 = property on="XY Graph" class="XYGraph (strict)"("ActYScl"=0 ("Active Y Scale")) -> ("YScale.Mapping Mode"=w328:u8)  [unwired: 2 in, 2 out]
                n244 = property on="XY Graph" class="XYGraph (strict)"("ActYScl"=1 ("Active Y Scale")) -> ("YScale.Mapping Mode"=w315:u8)  [unwired: 2 in, 2 out]
                n245 = Equal To 0?(x=w328) -> (x = 0?=w322:bool)
                n246 = Equal To 0?(x=w315) -> (x = 0?=w321:bool)
                n247 = Select(t=u8 1, s=w322, f=u8 0) -> (s? t:f=w325:u8)
                n248 = Select(t=u8 1, s=w321, f=u8 0) -> (s? t:f=w318:u8)
                n249 = property on="XY Graph" class="XYGraph (strict)"("ActYScl"=0 ("Active Y Scale"), "YScale.Mapping Mode"=w325) -> ()  [unwired: 2 in, 2 out]
                n250 = property on="XY Graph" class="XYGraph (strict)"("ActYScl"=1 ("Active Y Scale"), "YScale.Mapping Mode"=w318) -> ()  [unwired: 2 in, 2 out]
              }
            }
            n251 = case shown="\"DA_SCALE_X_A\", \"DA_SCALE_Y_A\"" w250 {
              frame Default {
              }
              frame "DA_SCALE_X_A", "DA_SCALE_Y_A" {
                n252 = property on="ToolbarUpdate" class="Bool (strict)"("Val(Sgnl)"=TRUE ("Value (Signaling)")) -> ()  [unwired: 2 in, 2 out]
              }
            }
          }
          frame "DA_EXPORT_EXCEL" {
            w331 = enum16{"Curves", "Values", "Results", "WFM"}."Curves" ("Type")
            n253 = control-ref of="Legend"() -> (w330:refnum<vi>)
            n254 = call "CRYGet Graph Data in Graph.vi"("Legend Refnum"=w330, "Type In"=w331) -> ("Rows"=w332:i32[])  [unwired: 2 in, 7 out]
            n255 = call "CRYExport to Excel.vi"("Rows"=w332, "Type"=w331) -> ()  [unwired: 2 in, 8 out]
          }
          frame "DA_AXIS_MAG_HIDE", "DA_AXIS_MAG_VIEW" {
            n256 = local read "MagnitudeShow"() -> (w333:bool)
            n257 = local read "PhaseShow"() -> (w336:bool)
            n258 = Equal?(x="DA_AXIS_MAG_VIEW", y=w337) -> (x = y?=w334:bool)
            n259 = Compound Arithmetic op=AND(w333, invert w336) -> (w335:bool)
            n260 = case shown="True" w335 {
              tunnel: w334 -> [w339 _]
              frame False {
                n261 = flat-sequence {
                  tunnel: [w346] -> w342
                  tunnel: w339 -> [w345]
                  tunnel: [w343] -> w341
                  tunnel: w342 -> [w348]
                  tunnel: w341 -> [w347]
                  tunnel: [w347] -> w340
                  tunnel: w340 -> [w357]
                  frame #0 {
                    n262 = local write "MagnitudeShow"(w345) -> ()
                    n263 = control-ref of="This VI"() -> (w343:refnum<vi>)
                    n264 = local write "XY Graph"(cluster{"XY Graph":cluster{dbl, dbl}[]}[] [] ("XY Graph")) -> ()
                    n265 = call "CRYGet Graph Data.vi"("pGraph VI"=w343) -> ("Rows"=w346:i32[])  [unwired: 2 in, 8 out]
                  }
                  frame #1 {
                    n266 = call "CRYGet Two Units Rows.vi"("pGraph VI In"=w347, "Old Rows In"=w348) -> ("All Rows Out"=w351:i32[])  [unwired: 3 in, 6 out]
                    n267 = call "CRYPlot XY Graph.vi"("sOption"="Update", "pGraph VI In"=w347, "Selected Rows In"=w351) -> ("Color Info"=w354:u32[], "Curve Name"=w355:string[], "All Rows Out"=w349:i32[], "ItemSyms"=w353:i32[])  [unwired: 3 in, 2 out]
                    n268 = call "CRYData View Legend New Insert.vi"("Item Symbols"=w353, "Color Array"=w354, "ItemName Array"=w355, "pGraph VI In"=w347) -> ()  [unwired: 1 in, 7 out]
                    n269 = call "CRYSymbol Conversion.vi"("nDatas"=w349, "sActin"="ACTIVE") -> ()  [unwired: 10 in]
                  }
                  frame #2 {
                    n270 = call "CRYGet Boolean Reference.vi"("Label Name"="CursorPlot", "VI Refnum"=w357) -> ("Boolean Ref"=w360:refnum<vi>)  [unwired: 7 in, 2 out]
                    n271 = property on="AxisChange" class="Bool (strict)"("Val(Sgnl)"=TRUE ("Value (Signaling)")) -> ()  [unwired: 2 in, 2 out]
                    n272 = property class="Bool"(reference=w360, "Val(Sgnl)"=TRUE) -> ()  [unwired: 1 in, 2 out]
                  }
                }
              }
              frame True {
              }
            }
          }
          frame "DA_AXIS_PHA_HIDE", "DA_AXIS_PHA_VIEW" {
            n273 = local read "MagnitudeShow"() -> (w361:bool)
            n274 = local read "PhaseShow"() -> (w364:bool)
            n275 = Equal?(x="DA_AXIS_PHA_VIEW", y=w365) -> (x = y?=w362:bool)
            n276 = Compound Arithmetic op=AND(invert w361, w364) -> (w363:bool)
            n277 = case shown="True" w363 {
              tunnel: w362 -> [w367 _]
              frame False {
                n278 = flat-sequence {
                  tunnel: [w374] -> w370
                  tunnel: w367 -> [w371]
                  tunnel: [w372] -> w369
                  tunnel: w370 -> [w378]
                  tunnel: w369 -> [w379]
                  tunnel: [w379] -> w368
                  tunnel: w368 -> [w385]
                  frame #0 {
                    n279 = local write "PhaseShow"(w371) -> ()
                    n280 = control-ref of="This VI"() -> (w372:refnum<vi>)
                    n281 = local write "XY Graph"(cluster{"XY Graph":cluster{dbl, dbl}[]}[] [] ("XY Graph")) -> ()
                    n282 = call "CRYGet Graph Data.vi"("pGraph VI"=w372) -> ("Rows"=w374:i32[])  [unwired: 2 in, 8 out]
                  }
                  frame #1 {
                    n283 = call "CRYGet Two Units Rows.vi"("pGraph VI In"=w379, "Old Rows In"=w378) -> ("All Rows Out"=w377:i32[])  [unwired: 3 in, 6 out]
                    n284 = call "CRYPlot XY Graph.vi"("sOption"="Update", "pGraph VI In"=w379, "Selected Rows In"=w377) -> ("Color Info"=w382:u32[], "Curve Name"=w383:string[], "All Rows Out"=w375:i32[], "ItemSyms"=w381:i32[])  [unwired: 3 in, 2 out]
                    n285 = call "CRYData View Legend New Insert.vi"("Item Symbols"=w381, "Color Array"=w382, "ItemName Array"=w383, "pGraph VI In"=w379) -> ()  [unwired: 1 in, 7 out]
                    n286 = call "CRYSymbol Conversion.vi"("nDatas"=w375, "sActin"="ACTIVE") -> ()  [unwired: 10 in]
                  }
                  frame #2 {
                    n287 = call "CRYGet Boolean Reference.vi"("Label Name"="CursorPlot", "VI Refnum"=w385) -> ("Boolean Ref"=w388:refnum<vi>)  [unwired: 7 in, 2 out]
                    n288 = property on="AxisChange" class="Bool (strict)"("Val(Sgnl)"=TRUE ("Value (Signaling)")) -> ()  [unwired: 2 in, 2 out]
                    n289 = property class="Bool"(reference=w388, "Val(Sgnl)"=TRUE) -> ()  [unwired: 1 in, 2 out]
                  }
                }
              }
              frame True {
              }
            }
          }
          frame Default {
            n290 = Search/Split String(string=w397, search string/char (-)="#") -> (substring before match=w392:string, match + rest of string=w395:string)  [unwired: 2 out]
            n291 = call "CRYPreUpdate Sequence.vi"("EventName"="CurLibUpdate") -> ()  [unwired: 15 in]
            n292 = Decimal String To Number(string=w395, offset=1) -> (number=w393:i32)  [unwired: 2 out]
            n293 = case shown="0, Default" w393 {
              selector: w393 -> [_ w410]
              tunnel: w392 -> [w401 w412]
              tunnel: w391 -> [_ _]
              tunnel: w389 -> [w407 w408]
              frame 0, Default {
                n294 = Equal?(x="DA_EXPORT_DOCUMENT" ("y"), y=w401) -> (x = y?=w404:bool)
                n295 = Select(t="ADD_DOC", s=w404, f=w401) -> (s? t:f=w402:string)
                n296 = local read "GraphType"() -> (w399:string)
                n297 = local read "Graph Number"() -> (w405:i32)
                n298 = Format Into String(w402, w399, w405, 0 ("input 4")) -> (resulting string=w406:string)  [unwired: 3 in, 1 out]
                n299 = Enqueue Element(queue=w407, element=w406) -> ()  [unwired: 1 in, 4 out]
              }
              frame 1..10 {
                n300 = flat-sequence {
                  tunnel: w412 -> [w415]
                  tunnel: [w415] -> w411
                  tunnel: w410 -> [w414]
                  tunnel: [w413] -> w409
                  tunnel: w411 -> [w419]
                  tunnel: w409 -> [w417]
                  tunnel: w408 -> [w416]
                  frame #0 {
                    n301 = call "CRYSet Graph Cluster Data.vi"("Graph Number"=w414) -> ("DataType"=w413:string)  [unwired: 2 in, 8 out]
                  }
                  frame #1 {
                    n302 = local read "Graph Number"() -> (w418:i32)
                    n303 = Format Into String(w419, w417, w418, 0 ("input 3")) -> (resulting string=w421:string)  [unwired: 3 in, 1 out]
                    n304 = Enqueue Element(queue=w416, element=w421) -> ()  [unwired: 1 in, 4 out]
                  }
                }
              }
            }
          }
          frame "DA_PRE_HIDE", "DA_PRE_VIEW" {
            n305 = disable-structure shown="Disabled" {
              disable-tunnel: w422 -> [w424 _]
              frame Disabled {
                n306 = control-ref of="This VI"() -> (w425:refnum<vi>)
                n307 = call "CRYPreview InsDel.vi"(9:"XY" ("sOption"), "Graph VI Ref"=w425, "sAction"=w424) -> ()  [unwired: 9 in]
              }
              frame Enabled {
              }
            }
          }
          frame "DA_PAL_HIDE", "DA_PAL_VIEW" {
            n308 = Equal?(x="DA_PAL_VIEW" ("y"), y=w427) -> (x = y?=w426:bool)
            n309 = property on="PaletteShow" class="Bool (strict)"("Val(Sgnl)"=w426) -> ()  [unwired: 2 in, 2 out]
          }
          frame "DA_REMOVEALL" {
            n310 = property on="RemoveAll" class="Bool (strict)"("Val(Sgnl)"=TRUE ("Value (Signaling)")) -> ()  [unwired: 2 in, 2 out]
          }
        }
      }
      event Shortcut Menu Activation? {
        n311 = event-data() -> ("MenuRef"=w432:refnum<k9>, "Coords"=w433:T1)  [unwired: 6 out]
        n312 = local read "LegendShow"() -> (w430:bool)
        n313 = case shown="True" w430 {
          tunnel: w433 -> [_ w449]
          tunnel: w432 -> [_ w447]
          tunnel: w431 -> [_ w442]
          frame False {
          }
          frame True {
            n314 = invoke on="Legend" class="MCListbox (strict)" method="Point To Row Column"("Point"=w449) -> ("CellPosition"=w450:T5)  [unwired: 6 in, 6 out]
            n315 = local read "TotalPlot"() -> (w440:u32)
            n316 = control-ref of="Legend"() -> (w437:refnum<vi>)
            n317 = Unbundle By Name(w450) -> ("Row"=w436:i32)
            n318 = To Long Integer(number=w440) -> (32bit integer=w439:i32)
            n319 = Less?(x=w436, y=w439) -> (x < y?=w444:bool)
            n320 = local write "OldRow"(w436) -> ()
            n321 = Greater?(x=w440, y=u32 0) -> (0:w443:bool)
            n322 = local read "LegendVScrollShow"() -> (w434:bool)
            n323 = local read "LegendShow"() -> (w445:bool)
            n324 = call "CRYGet Selected Data in Legend.vi"("Right Clicked Row"=w436, "Legend Ref"=w437) -> ("Selected Rows"=w435:i32[])  [unwired: 9 in]
            n325 = local write "SelectedRow"(w435) -> ()
            n326 = property on="Legend" class="MCListbox (strict)"("Value"=w435) -> ()  [unwired: 2 in, 2 out]
            n327 = Bundle By Name(cluster=w442, "LegendShow"=w445, "CellClick"=w444, "Total Number"=w443, "LegendVScrollShow"=w434) -> (w441:T2)
            n328 = control-ref of="This VI"() -> (w438:refnum<vi>)
            n329 = call "CRYGraph Window Menu.vi"("pGraph VI"=w438, "Flag Cluster"=w441, "Type"="LEGEND", "Runtime Menu Ref In"=w447) -> ()  [unwired: 1 in, 7 out]
          }
        }
        n330 = event-data() -> ()  [unwired: 1 in, 2 out]
      }
      event Shortcut Menu Selection (User) {
        n331 = event-data() -> ("ItemTag"=w455:string)  [unwired: 8 out]
        n332 = local read "Graph Number"() -> (w452:i32)
        n333 = case shown="\"DA_LEG_REMOVEALL\"" w455 {
          selector: w455 -> [_ _ _ _ _ _ w488]
          tunnel: w454 -> [_ w460 _ _ _ _ _]
          tunnel: w452 -> [_ w459 _ _ _ _ _]
          tunnel: w451 -> [_ w457 _ _ _ _ _]
          frame Default {
          }
          frame "DA_LEG_HIDE_1" {
            n334 = Format Into String("DA_LEG_HIDE" ("input 1"), w457, w459, 0 ("input 3")) -> (resulting string=w461:string)  [unwired: 3 in, 1 out]
            n335 = Enqueue Element(queue=w460, element=w461) -> ()  [unwired: 1 in, 4 out]
          }
          frame "DA_LEG_REMOVE" {
            n336 = property on="RemoveSome" class="Bool (strict)"("Val(Sgnl)"=TRUE ("Value (Signaling)")) -> ()  [unwired: 2 in, 2 out]
          }
          frame "DA_LEG_REMOVEALL" {
            n337 = property on="RemoveAll" class="Bool (strict)"("Val(Sgnl)"=TRUE ("Value (Signaling)")) -> ()  [unwired: 2 in, 2 out]
          }
          frame "DA_LEG_INVERT" {
            n338 = local read "TotalPlot"() -> (w465:u32)
            n339 = for {
              N: w465 -> [_]
              tunnel: [w469] -> w466
              tunnel: [w468] -> w464
              i -> [w471]
              w473 = 38
              w475 = 37
              n340 = property on="Legend" class="MCListbox (strict)"() -> ("ItemSyms"=w477:i32[])  [unwired: 2 in, 2 out]
              n341 = Index Array(array=w477, index=w471) -> (element=w476:i32)
              n342 = To Unsigned Long Integer(number=w471) -> (unsigned 32bit integer=w470:u32)
              n343 = Equal?(x=w476, y=w475) -> (x = y?=w472:bool)
              n344 = Equal?(x=w476, y=w473) -> (x = y?=w474:bool)
              n345 = Select(t=w475, s=w474, f=w473) -> (s? t:f=w478:i32)
              n346 = Replace Array Subset(array=w477, new element=w478, index=w471) -> (w479:i32[])
              n347 = property on="XY Graph" class="XYGraph (strict)"("Active Plot"=w470, "Plot.Visible?"=w472) -> (error out=w468:errorcluster)  [unwired: 2 in, 1 out]
              n348 = property on="Legend" class="MCListbox (strict)"("ItemSyms"=w479) -> (error out=w469:errorcluster)  [unwired: 2 in, 1 out]
            }
            n349 = case shown="No Error" w464 {
              frame No Error {
              }
              frame Error {
              }
            }
            n350 = property on="AxisChange" class="Bool (strict)"(error in=w466, "Val(Sgnl)"=TRUE ("Value (Signaling)")) -> ()  [unwired: 1 in, 2 out]
          }
          frame "DA_LEG_SHOWALL" {
            n351 = local read "TotalPlot"() -> (w480:u32)
            n352 = for {
              N: w480 -> [_]
              tunnel: [38] -> w483 mode=indexing
              i -> [w487]
              n353 = To Unsigned Long Integer(number=w487) -> (unsigned 32bit integer=w486:u32)
              n354 = property on="XY Graph" class="XYGraph (strict)"("Active Plot"=w486, "Plot.Visible?"=TRUE ("Plot.Visible")) -> ()  [unwired: 2 in, 2 out]
            }
            n355 = property on="Legend" class="MCListbox (strict)"("ItemSyms"=w483) -> (error out=w482:errorcluster)  [unwired: 2 in, 1 out]
            n356 = property on="AxisChange" class="Bool (strict)"(error in=w482, "Val(Sgnl)"=TRUE ("Value (Signaling)")) -> ()  [unwired: 1 in, 2 out]
          }
          frame "DA_LEG_VSCROLL_HIDE", "DA_LEG_VSCROLL_VIEW" {
            n357 = Equal?(x="DA_LEG_VSCROLL_VIEW" ("y"), y=w488) -> (x = y?=w489:bool)
            n358 = property on="LegendVScrollShow" class="Bool (strict)"("Val(Sgnl)"=w489) -> ()  [unwired: 2 in, 2 out]
          }
        }
        n359 = call "CRYPreUpdate Sequence.vi"("EventName"="CurLibUpdate") -> ()  [unwired: 15 in]
      }
      event Shortcut Menu Activation? {
        n360 = event-data() -> ("MenuRef"=w493:refnum<k9>)  [unwired: 7 out]
        n361 = local read "CursorShow"() -> (w491:bool)
        n362 = case shown="True" w491 {
          selector: w491 -> [_ w494]
          tunnel: w493 -> [_ w497]
          tunnel: w492 -> [_ w496]
          frame False {
          }
          frame True {
            n363 = Bundle By Name(cluster=w496, "CursorShow"=w494) -> (w498:T2)
            n364 = control-ref of="This VI"() -> (w495:refnum<vi>)
            n365 = call "CRYGraph Window Menu.vi"("pGraph VI"=w495, "Flag Cluster"=w498, "Type"="CURSOR", "Runtime Menu Ref In"=w497) -> ()  [unwired: 1 in, 7 out]
          }
        }
        n366 = event-data() -> ()  [unwired: 2 in, 1 out]
      }
      event Shortcut Menu Selection (User) {
        n367 = event-data() -> ("ItemTag"=w502:string)  [unwired: 8 out]
        n368 = local read "Graph Number"() -> (w504:i32)
        n369 = Match Pattern(string=w502, regular expression="#" ("search string/char (-)")) -> (before substring=w501:string, after substring=w500:string)  [unwired: 1 in, 2 out]
        n370 = case shown="\"LINKTO\"" w501 {
          selector: w501 -> [_ _ _ w539 _]
          tunnel: w507 -> [_ _ _ w537 w544]
          tunnel: w504 -> [_ _ _ w540 w546]
          tunnel: w506 -> [_ _ _ w538 w545]
          tunnel: w500 -> [w508 _ w523 _ _]
          frame "DA_CUR_GOTO_CUR" {
            n371 = Decimal String To Number(string=w508) -> (number=w509:i32)  [unwired: 1 in, 2 out]
            n372 = case shown="0, 1" w509 {
              selector: w509 -> [_ w511]
              frame Default {
              }
              frame 0, 1 {
                n373 = flat-sequence {
                  tunnel: w511 -> [w513]
                  frame #0 {
                    n374 = Equal To 0?(x=w513) -> (x = 0?=w517:bool)
                    n375 = local write "NewCursIdx"(w513) -> ()
                    n376 = property on="XY Graph" class="XYGraph (strict)"("Active Cursor"=w513) -> ()  [unwired: 2 in, 2 out]
                    n377 = Select(t=1 ("OldCursIdx"), s=w517, f=0 ("OldCursIdx")) -> (s? t:f=w514:i32)
                    n378 = local write "OldCursIdx"(w514) -> ()
                  }
                  frame #1 {
                    n379 = property on="CursorColor" class="Bool (strict)"("Val(Sgnl)"=TRUE ("Value (Signaling)")) -> ()  [unwired: 2 in, 2 out]
                  }
                }
                n380 = control-ref of="XY Graph"() -> (w510:refnum<vi>)
                n381 = call "CRYGoto Cursor.vi"("Active Cursor"=w511, "Graph Ref"=w510, "Graph Type"="XY") -> ()  [unwired: 9 in]
              }
            }
          }
          frame "DA_BRING_CENTER" {
            n382 = property on="XY Graph" class="XYGraph (strict)"() -> ("Active Cursor"=w519:u32)  [unwired: 2 in, 2 out]
            n383 = control-ref of="XY Graph"() -> (w521:refnum<vi>)
            n384 = call "CRYGoto Cursor.vi"("sOption"="Bring_to_Center", "Active Cursor"=w519, "Graph Ref"=w521, "Graph Type"="XY") -> ()  [unwired: 8 in]
          }
          frame "LINKTO" {
            n385 = Match Pattern(string=w523, regular expression="[0-1]_") -> (match substring=w527:string, after substring=w525:string)  [unwired: 1 in, 2 out]
            n386 = Decimal String To Number(string=w527) -> (number=w524:i32)  [unwired: 2 in, 1 out]
            n387 = case shown="0, 1" w524 {
              selector: w524 -> [w528 _]
              tunnel: w525 -> [w529 _]
              frame 0, 1 {
                n388 = control-ref of="Legend"() -> (w531:refnum<vi>)
                n389 = call "CRYGet Legend Name.vi"("MCListbox Refnum"=w531) -> ("Names Out"=w532:string[])  [unwired: 10 in]
                n390 = control-ref of="XY Graph"() -> (w530:refnum<vi>)
                n391 = Search 1D Array(1D array=w532, element=w529) -> (index of element=w533:i32)  [unwired: 1 in]
                n392 = case shown="-1" w533 {
                  selector: w533 -> [w535 _]
                  tunnel: w530 -> [w536 _]
                  tunnel: w528 -> [w534 _]
                  frame 0, Default {
                    n393 = property class="XYGraph (strict)"(reference=w536, "Active Cursor"=w534, "Cursor.Cursor Plot"=w535) -> ()  [unwired: 1 in, 2 out]
                  }
                  frame -1 {
                  }
                }
              }
              frame Default {
              }
            }
          }
          frame Default {
            n394 = Format Into String(w539, w538, w540, 0 ("input 3")) -> (resulting string=w541:string)  [unwired: 3 in, 1 out]
            n395 = Enqueue Element(queue=w537, element=w541) -> ()  [unwired: 1 in, 4 out]
          }
          frame "DA_CUR_HIDE_1" {
            n396 = Format Into String("DA_CUR_HIDE", w545, w546, 0 ("input 3")) -> (resulting string=w547:string)  [unwired: 3 in, 1 out]
            n397 = Enqueue Element(queue=w544, element=w547) -> ()  [unwired: 1 in, 4 out]
          }
        }
        n398 = call "CRYPreUpdate Sequence.vi"("EventName"="CurLibUpdate") -> ()  [unwired: 15 in]
      }
      event Shortcut Menu Activation? {
        n399 = event-data() -> ("MenuRef"=w549:refnum<k9>)  [unwired: 7 out]
        n400 = disable-structure shown="Disabled" {
          disable-tunnel: w550 -> [w553 _]
          disable-tunnel: w549 -> [w552 _]
          frame Disabled {
            n401 = local read "PreviewShow"() -> (w551:bool)
            n402 = case shown="True" w551 {
              selector: w551 -> [_ w554]
              tunnel: w553 -> [_ w556]
              tunnel: w552 -> [_ w555]
              frame False {
              }
              frame True {
                n403 = Bundle By Name(cluster=w556, "PreviewShow"=w554) -> (w558:T2)
                n404 = control-ref of="This VI"() -> (w557:refnum<vi>)
                n405 = call "CRYGraph Window Menu.vi"("pGraph VI"=w557, "Flag Cluster"=w558, "Type"="PREVIEW", "Runtime Menu Ref In"=w555) -> ()  [unwired: 1 in, 7 out]
              }
            }
          }
          frame Enabled {
          }
        }
        n406 = event-data() -> ()  [unwired: 2 in, 1 out]
      }
      event Shortcut Menu Selection (User) {
        n407 = event-data() -> ("ItemTag"=w560:string)  [unwired: 8 out]
        n408 = disable-structure shown="Disabled" {
          disable-tunnel: w560 -> [w561 _]
          frame Disabled {
            n409 = case shown="\"DA_PRE_LOCATION\"" w561 {
              frame Default {
              }
              frame "DA_PRE_SHOWALL" {
                n410 = flat-sequence {
                  frame #0 {
                    w565 = u8 2 ("X Scale.Scale Fit")
                    n411 = property on="XY Graph" class="XYGraph (strict)"("XScale.ScaleFit"=w565, "ActYScl"=0 ("Active Y Scale"), "YScale.ScaleFit"=w565, "ActYScl"=1 ("Active Y Scale"), "YScale.ScaleFit"=w565) -> ()  [unwired: 2 in, 2 out]
                    n412 = property on="PreviewGraph" class="XYGraph (strict)"("XScale.ScaleFit"=w565) -> (error out=w562:errorcluster)  [unwired: 2 in, 1 out]
                    n413 = property on="PreviewGraph" class="XYGraph (strict)"(error in=w562) -> ("XScale.Maximum"=w564:dbl, "XScale.Minimum"=w563:dbl)  [unwired: 1 in, 2 out]
                    n414 = property on="XY Graph" class="XYGraph (strict)"("XScale.Maximum"=w564, "XScale.Minimum"=w563) -> ()  [unwired: 2 in, 2 out]
                  }
                  frame #1 {
                    n415 = property on="ScaleRange" class="Bool (strict)"("Val(Sgnl)"=TRUE ("Value (Signaling)")) -> ()  [unwired: 2 in, 2 out]
                  }
                }
              }
              frame "DA_PRE_LOCATION" {
                n416 = flat-sequence {
                  frame #0 {
                    w569 = u8 0 ("X Scale.Scale Fit")
                    n417 = property on="Scrollbar" class="Scroll (strict)"() -> ("PageSize"=w574:dbl, "Value"=w573:dbl)  [unwired: 2 in, 2 out]
                    n418 = local read "PreviewCoords"() -> (w593:T1)
                    n419 = property on="PreviewGraph" class="XYGraph (strict)"() -> ("Plot Bounds"=w597:T6, "Width"=w596:u32)  [unwired: 2 in, 2 out]
                    n420 = Equal?(x=w574, y=w573) -> (x = y?=w572:bool)
                    n421 = property on="XY Graph" class="XYGraph (strict)"("XScale.ScaleFit"=w569, "ActYScl"=0 ("Active Y Scale"), "YScale.ScaleFit"=w569, "ActYScl"=1 ("Active Y Scale"), "YScale.ScaleFit"=w569) -> ()  [unwired: 2 in, 2 out]
                    n422 = case shown="True" w572 {
                      tunnel: [w605 w610] -> w592
                      frame False {
                        n423 = property on="PreviewGraph" class="XYGraph (strict)"("Active Cursor"=u32 0, "Active Cursor"=u32 1) -> ("Cursor.Cursor X"=w603:dbl, "Cursor.Cursor X"=w604:dbl)  [unwired: 2 in, 2 out]
                        n424 = Greater?(x=w603, y=w604) -> (0:w602:bool)
                        n425 = case shown="True" w602 {
                          tunnel: w603 -> [w607 w609]
                          tunnel: w604 -> [w606 w608]
                          tunnel: [w607 w608] -> w598
                          tunnel: [w606 w609] -> w599
                          frame False {
                          }
                          frame True {
                          }
                        }
                        n426 = Subtract(x=w599, y=w598) -> (x-y=w605:dbl)
                      }
                      frame True {
                        n427 = property on="PreviewGraph" class="XYGraph (strict)"("ActXScl"=0 ("Active X Scale")) -> ("XScale.Maximum"=w614:dbl, "XScale.Minimum"=w613:dbl)  [unwired: 2 in, 2 out]
                        n428 = Subtract(x=w614, y=w613) -> (x-y=w612:dbl)
                        n429 = Divide(x=w612, y=20.0) -> (x/y=w610:dbl)
                      }
                    }
                    n430 = Unbundle By Name(w593) -> ("Horizontal"=w586:i32)
                    n431 = To Long Integer(number=w596) -> (32bit integer=w581:i32)
                    n432 = Unbundle By Name(w597) -> ("Left"=w595:i16)
                    n433 = property on="PreviewGraph" class="XYGraph (strict)"("XScale.ScaleFit"=w569) -> ()  [unwired: 2 in, 2 out]
                    n434 = To Long Integer(number=w595) -> (32bit integer=w584:i32)
                    n435 = Add(x=w584, y=w581) -> (x+y=w594:i32)
                    n436 = Less?(x=w586, y=w584) -> (x < y?=w590:bool)
                    n437 = Greater?(x=w586, y=w594) -> (0:w589:bool)
                    n438 = property on="PreviewGraph" class="XYGraph (strict)"("ActXScl"=0 ("Active X Scale")) -> ("XScale.Maximum"=w577:dbl, "XScale.Minimum"=w579:dbl)  [unwired: 2 in, 2 out]
                    n439 = Build Array(w590, w589) -> (w588:bool[])
                    n440 = Search 1D Array(1D array=w588, element=TRUE) -> (index of element=w583:i32)  [unwired: 1 in]
                    n441 = Divide(x=w592, y=2.0) -> (x/y=w585:dbl)
                    n442 = Subtract(x=w577, y=w579) -> (x-y=w580:dbl)
                    n443 = case shown="Default" w583 {
                      tunnel: w586 -> [_ _ w630]
                      tunnel: [w616 w620 w622] -> w578
                      tunnel: w585 -> [w618 w621 _]
                      tunnel: w584 -> [_ _ w629]
                      tunnel: w581 -> [_ _ w627]
                      tunnel: w580 -> [_ _ w625]
                      tunnel: w579 -> [w617 _ w623]
                      tunnel: w577 -> [_ w619 _]
                      frame 0 {
                        n444 = Add(x=w618, y=w617) -> (x+y=w616:dbl)
                      }
                      frame 1 {
                        n445 = Subtract(x=w619, y=w621) -> (x-y=w620:dbl)
                      }
                      frame Default {
                        n446 = Subtract(x=w630, y=w629) -> (x-y=w628:i32)
                        n447 = Divide(x=w628, y=w627) -> (x/y=w626:dbl)
                        n448 = Multiply(x=w626, y=w625) -> (x*y=w624:dbl)
                        n449 = Add(x=w624, y=w623) -> (x+y=w622:dbl)
                      }
                    }
                    n450 = Add(x=w578, y=w585) -> (x+y=w576:dbl)
                    n451 = Subtract(x=w578, y=w585) -> (x-y=w575:dbl)
                    n452 = property on="XY Graph" class="XYGraph (strict)"("XScale.Maximum"=w576, "XScale.Minimum"=w575) -> ()  [unwired: 2 in, 2 out]
                  }
                  frame #1 {
                    n453 = property on="ScaleRange" class="Bool (strict)"("Val(Sgnl)"=TRUE ("Value (Signaling)")) -> ()  [unwired: 2 in, 2 out]
                  }
                }
              }
              frame "DA_PRE_HIDE_1" {
                n454 = property on="PreviewShow" class="Bool (strict)"("Val(Sgnl)"=FALSE ("Value (Signaling)")) -> ()  [unwired: 2 in, 2 out]
              }
            }
          }
          frame Enabled {
          }
        }
      }
      event "PaletteShow": Value Change {
        n455 = event-data() -> ("NewVal"=w633:bool)  [unwired: 6 out]
        n456 = property on="XY Graph" class="XYGraph (strict)"("Palette Visible"=w633) -> ()  [unwired: 2 in, 2 out]
      }
      event "Cursor": Key Down {
        n457 = event-data() -> ("ScanCode"=w635:i16)  [unwired: 10 out]
        n458 = case shown="75, 77" w635 {
          selector: w635 -> [_ w637]
          tunnel: w634 -> [_ w638]
          frame Default {
          }
          frame 75, 77 {
            n459 = flat-sequence {
              tunnel: w637 -> [w641]
              tunnel: [w641] -> w636
              tunnel: w638 -> [w650]
              tunnel: w636 -> [w647]
              frame #0 {
                n460 = local write "CursorMoveFinish"(TRUE ("CursorMove")) -> ()
                n461 = local write "KeyRepeatCount"(1 ("KeyRepeatCount")) -> ()
              }
              frame #1 {
                n462 = Equal?(x=i16 75, y=w647) -> (x = y?=w643:bool)
                n463 = Select(t="Left" ("input 2"), s=w643, f="Right" ("input 2")) -> (s? t:f=w642:string)
                n464 = To Long Integer(number=w647) -> (32bit integer=w649:i32)
                n465 = local write "WhichKey"(w642) -> ()
                n466 = Format Into String("Cursor_Move" ("input 1"), w642, w649, 0 ("input 4")) -> (resulting string=w651:string)  [unwired: 3 in, 1 out]
                n467 = Enqueue Element(queue=w650, element=w651) -> ()  [unwired: 1 in, 4 out]
              }
            }
          }
        }
      }
      event "Cursor": Key Repeat {
        n468 = event-data() -> ("ScanCode"=w654:i16)  [unwired: 10 out]
        n469 = case shown="75, 77" w654 {
          selector: w654 -> [_ w656]
          tunnel: w653 -> [_ w657]
          frame Default {
          }
          frame 75, 77 {
            n470 = flat-sequence {
              tunnel: w656 -> [w660]
              tunnel: [w660] -> w655
              tunnel: w657 -> [w665]
              tunnel: w655 -> [w663]
              frame #0 {
                n471 = local read "KeyRepeatCount"() -> (w659:i32)
                n472 = Increment(x=w659) -> (x+1=w658:i32)
                n473 = local write "KeyRepeatCount"(w658) -> ()
              }
              frame #1 {
                n474 = local read "WhichKey"() -> (w661:string)
                n475 = To Long Integer(number=w663) -> (32bit integer=w664:i32)
                n476 = Format Into String("Cursor_Move" ("input 1"), w661, w664, 0 ("input 4")) -> (resulting string=w666:string)  [unwired: 3 in, 1 out]
                n477 = Enqueue Element(queue=w665, element=w666) -> ()  [unwired: 1 in, 4 out]
              }
            }
          }
        }
      }
      event "Cursor": Key Up {
        n478 = event-data() -> ("ScanCode"=w669:i16)  [unwired: 8 out]
        n479 = case shown="75, 77" w669 {
          selector: w669 -> [_ w671]
          tunnel: w668 -> [_ w672]
          frame Default {
          }
          frame 75, 77 {
            n480 = flat-sequence {
              tunnel: w671 -> [w674]
              tunnel: [w674] -> w670
              tunnel: w672 -> [w683]
              tunnel: w670 -> [w679]
              frame #0 {
                n481 = local write "CursorMoveFinish"(FALSE ("CursorMoveFinish")) -> ()
              }
              frame #1 {
                n482 = Equal?(x=i16 75, y=w679) -> (x = y?=w678:bool)
                n483 = Select(t="Left" ("input 2"), s=w678, f="Right" ("input 2")) -> (s? t:f=w675:string)
                n484 = To Long Integer(number=w679) -> (32bit integer=w682:i32)
                n485 = local write "WhichKey"(w675) -> ()
                n486 = Format Into String("Cursor_Move" ("input 1"), w675, w682, 0 ("input 4")) -> (resulting string=w684:string)  [unwired: 3 in, 1 out]
                n487 = Enqueue Element(queue=w683, element=w684) -> ()  [unwired: 1 in, 4 out]
              }
            }
          }
        }
      }
      event "Cursor": Mouse Down {
        n488 = event-data() -> ("CtlRef"=w689:refnum<vi>, "Coords"=w686:T1)  [unwired: 7 out]
        n489 = local write "Cursor Coords"(w686) -> ()
        n490 = invoke class="Tbl (strict)" method="Point To Row Column"(reference=w689, "Point"=w686) -> ("CellPosition"=w688:T5)  [unwired: 4 in, 5 out]
        n491 = Unbundle By Name(w688) -> ("Row"=w687:i32)
        n492 = flat-sequence {
          tunnel: w687 -> [w690]
          frame #0 {
            n493 = Equal To 0?(x=w690) -> (x = 0?=w694:bool)
            n494 = local write "NewCursIdx"(w690) -> ()
            n495 = property on="XY Graph" class="XYGraph (strict)"("Active Cursor"=w690) -> ()  [unwired: 2 in, 2 out]
            n496 = Select(t=1 ("OldCursIdx"), s=w694, f=0 ("OldCursIdx")) -> (s? t:f=w691:i32)
            n497 = local write "OldCursIdx"(w691) -> ()
          }
          frame #1 {
            n498 = property on="CursorColor" class="Bool (strict)"("Val(Sgnl)"=TRUE ("Value (Signaling)")) -> ()  [unwired: 2 in, 2 out]
          }
        }
      }
      event "Cursor": Value Change {
        n499 = event-data() -> ("OldVal"=w700:string[][], "NewVal"=w699:string[][])  [unwired: 5 out]
        n500 = local read "Cursor Coords"() -> (w697:T1)
        n501 = control-ref of="This VI"() -> (w698:refnum<vi>)
        n502 = call "CRYCursor move in Cursor Table.vi"("NewVal"=w699, "OldVal"=w700, "Cursor Coords"=w697, "pGraph VI"=w698) -> ("NewVal Out"=w696:string[][])  [unwired: 7 in]
        n503 = local write "Cursor"(w696) -> ()
      }
      event "CursorShow": Value Change {
        n504 = event-data() -> ("NewVal"=w701:bool)  [unwired: 6 out]
        n505 = flat-sequence {
          tunnel: w701 -> [w706]
          frame #0 {
            n506 = Select(t="DA_CUR_VIEW", s=w706, f="DA_CUR_HIDE") -> (s? t:f=w705:string)
            n507 = control-ref of="This VI"() -> (w702:refnum<vi>)
            n508 = call "CRYCursor InsDel.vi"("Graph VI Ref"=w702, "sAction"=w705) -> ()  [unwired: 10 in]
          }
          frame #1 {
            n509 = property on="ToolbarUpdate" class="Bool (strict)"("Val(Sgnl)"=TRUE ("Value (Signaling)")) -> ()  [unwired: 2 in, 2 out]
          }
        }
      }
      event "CursorPlot": Value Change {
        n510 = event-data() -> ()  [unwired: 7 out]
        n511 = local read "CursorShow"() -> (w708:bool)
        n512 = case shown="True" w708 {
          frame False {
          }
          frame True {
            n513 = control-ref of="XY Graph"() -> (w711:refnum<vi>)
            n514 = control-ref of="Cursor"() -> (w710:refnum<vi>)
            n515 = call "CRYPlot Cursor.vi"("Cursor Ref"=w710, "Graph Ref"=w711, "Graph Type"="XY") -> ()  [unwired: 9 in]
          }
        }
      }
      event "CursorColor": Value Change {
        n516 = event-data() -> ()  [unwired: 7 out]
        n517 = local read "NewCursIdx"() -> (w722:u32)
        n518 = local read "OldCursIdx"() -> (w723:u32)
        n519 = property on="XY Graph" class="XYGraph (strict)"("Active Cursor"=w723) -> ("Cursor.Cursor Color"=w715:u32)  [unwired: 2 in, 2 out]
        n520 = property on="XY Graph" class="XYGraph (strict)"("Active Cursor"=w722) -> ("Cursor.Cursor Color"=w714:u32)  [unwired: 2 in, 2 out]
        n521 = Bundle By Name(cluster=T5 {"Row"=0, "Column"=0} ("Active Cell:Active Cell"), "Row"=w722, "Column"=0) -> (w719:T5)
        n522 = Bundle By Name(cluster=T5 {"Row"=0, "Column"=0} ("Active Cell:Active Cell"), "Row"=w723, "Column"=0) -> (w716:T5)
        n523 = property on="Cursor" class="Tbl (strict)"("Active Cell"=w716, "CellFontColor"=w715, "Cell BG Color"=u32 16777226) -> ()  [unwired: 2 in, 2 out]
        n524 = property on="Cursor" class="Tbl (strict)"("Active Cell"=w719, "CellFontColor"=w714, "Cell BG Color"=u32 60927) -> ()  [unwired: 2 in, 2 out]
      }
      event "Legend": Mouse Down {
        n525 = event-data() -> ("CtlRef"=w725:refnum<vi>, "Coords"=w730:T1, "Button"=w729:u16)  [unwired: 6 out]
        n526 = local read "TotalPlot"() -> (w726:u32)
        n527 = call "CRYData View Legend Plot OnOff.vi"("TotalPlot"=w726, "Button Info"=w729, "Mouse Point"=w730, "MCListbox Ref In"=w725) -> ("Active Row"=w724:i32, "Visible?"=w727:bool, "Click State"=w728:bool)  [unwired: 5 out]
        n528 = case shown="True" w728 {
          tunnel: w727 -> [_ w736]
          tunnel: w724 -> [_ w737]
          frame False {
          }
          frame True {
            w732 = u8 0 ("Y Scale.Scale Fit")
            n529 = property on="PreviewGraph" class="XYGraph (strict)"("XScale.ScaleFit"=w732) -> ()  [unwired: 2 in, 2 out]
            n530 = property on="XY Graph" class="XYGraph (strict)"("XScale.ScaleFit"=w732) -> (error out=w733:errorcluster)  [unwired: 2 in, 1 out]
            n531 = property on="AxisChange" class="Bool (strict)"("Val(Sgnl)"=TRUE ("Value (Signaling)")) -> ()  [unwired: 2 in, 2 out]
            n532 = To Unsigned Long Integer(number=w737) -> (unsigned 32bit integer=w735:u32)
            n533 = property on="XY Graph" class="XYGraph (strict)"(error in=w733, "Active Plot"=w735, "Plot.Visible?"=w736) -> (error out=w731:errorcluster)  [unwired: 1 in, 1 out]
            n534 = case shown="No Error" w731 {
              frame No Error {
              }
              frame Error {
              }
            }
          }
        }
      }
      event "Legend": Double Click {
        n535 = event-data() -> ("CtlRef"=w739:refnum<vi>, "Coords"=w738:T1)  [unwired: 8 out]
        n536 = disable-structure shown="Disabled" {
          disable-tunnel: w739 -> [w745 _]
          disable-tunnel: w738 -> [w744 _]
          frame Disabled {
            n537 = call "CRYGet MultiListBox Click State.vi"("Coords"=w744, "MultiList Box Ref In"=w745) -> ("State"=w743:bool)  [unwired: 6 in, 3 out]
            n538 = call "CRYClick Name in Legend.vi"("Mouse Point"=w744, "MCListbox Ref In"=w745) -> ("Active Row"=w741:i32, "Click State?"=w742:bool)  [unwired: 8 in]
            n539 = And(x=w743, y=w742) -> (x .and. y?=w740:bool)
            n540 = case shown="True" w740 {
              tunnel: w745 -> [_ w746]
              tunnel: w741 -> [_ w747]
              frame False {
              }
              frame True {
                n541 = call "CRYOpen Step by Legend.vi"("Active Row"=w747, "MCListbox Ref In"=w746, "Type"=enum16{"Curves", "Values", "Results", "WFM"}."Curves" ("Type In")) -> ()  [unwired: 9 in]
              }
            }
          }
          frame Enabled {
          }
        }
      }
      event "Legend": Mouse Move {
        n542 = event-data() -> ("CtlRef"=w749:refnum<vi>, "Coords"=w756:T1)  [unwired: 4 out]
        n543 = local read "TotalPlot"() -> (w755:u32)
        n544 = call "CRYData View Legend Mouse Move.vi"("TotalPlot"=w755, "Mouse Point"=w756, "MCListbox Ref In"=w749) -> ("CellSize"=w753:T7, "Position"=w752:T8, "Selected Row"=w751:i32, "Move State"=w750:bool, "CellBG"=w754:u32)  [unwired: 1 in, 3 out]
        n545 = case shown="True" w750 {
          tunnel: w754 -> [_ w762]
          tunnel: w753 -> [_ w761]
          tunnel: w752 -> [_ w760]
          tunnel: w751 -> [_ w759]
          frame False {
            n546 = property on="ColorBox" class="ColBox"("Visible"=FALSE) -> ()  [unwired: 2 in, 2 out]
          }
          frame True {
            n547 = local write "OldRow"(w759) -> ()
            n548 = property on="ColorBox" class="ColBox"("Position"=w760, "Color Area Size"=w761, "Value"=w762, "Visible"=TRUE) -> ()  [unwired: 2 in, 2 out]
          }
        }
      }
      event "Legend": Value Change {
        n549 = event-data() -> ("NewVal"=w764:i32[])  [unwired: 6 out]
        n550 = local read "Test"() -> (w763:string)
        n551 = case shown="Default" w763 {
          tunnel: w764 -> [_ w768]
          frame "Test" {
          }
          frame Default {
            n552 = control-ref of="Legend"() -> (w770:refnum<vi>)
            n553 = local read "MagnitudeShow"() -> (w771:bool)
            n554 = local read "PhaseShow"() -> (w772:bool)
            n555 = call "CRYGet Legend Name.vi"("MCListbox Refnum"=w770) -> ("Names Out"=w769:string[])  [unwired: 10 in]
            n556 = Compound Arithmetic op=AND(w771, w772) -> (w766:bool)
            n557 = case shown="True" w766 {
              tunnel: w769 -> [_ w784]
              tunnel: w768 -> [w780 w783]
              tunnel: [w780 w781] -> w767
              frame False {
              }
              frame True {
                n558 = for {
                  tunnel: w784 -> [w797]
                  tunnel: w783 -> [w785] mode=indexing
                  shift-right: [w789] -> w781
                  shift-left: i32[] [] ("NewVal") -> [w790]
                  n559 = Index Array(array=w797, index=w785) -> (element=w791:string)
                  n560 = Match Pattern(string=w791, regular expression=" \\[Phase\\]") -> (after substring=w795:string, offset past match=w794:i32)  [unwired: 1 in, 2 out]
                  n561 = Empty String/Path?(string/path=w795) -> (empty?=w793:bool)
                  n562 = Greater Than 0?(x=w794) -> (x > 0?=w792:bool)
                  n563 = And(x=w793, y=w792) -> (x .and. y?=w788:bool)
                  n564 = Decrement(x=w785) -> (x-1=w787:i32)
                  n565 = Select(t=w787, s=w788, f=w785) -> (s? t:f=w786:i32)
                  n566 = Insert Into Array(array=w790, new element=w786) -> (w789:i32[])  [unwired: 1 in]
                }
              }
            }
            n567 = control-ref of="Legend"() -> (w777:refnum<vi>)
            n568 = local read "GraphType"() -> (w773:string)
            n569 = call "CRYData View Legend Manipulate.vi"("sAction"="GetViewNumbyLegNum", "nData"=w767, "sData"=w773, "Legend Ref"=w777) -> ("nData Out"=w774:i32[])  [unwired: 6 in, 1 out]
            n570 = call "CRYGet Graph Name From Graph Type.vi"("Graph Type"=w773) -> ("Type"=w776:enum16{"Curves", "Values", "Results", "WFM"})  [unwired: 9 in, 1 out]
            n571 = call "CRYTree Global Manipulate.vi"("Type In"=w776) -> ("Tree/Curve Tree"=w775:refnum<vi>)  [unwired: 7 in, 3 out]
            n572 = call "CRYTree Manuplate.vi"("sAction"="SetActiveNumbers", "nData"=w774, "Tree in"=w775) -> ("Tree Out"=w765:refnum<vi>)  [unwired: 5 in, 3 out]
            n573 = flat-sequence {
              tunnel: w765 -> [_]
              frame #0 {
                n574 = call "CRYUpdate Buttons.vi"() -> ()  [unwired: 12 in]
              }
            }
          }
        }
      }
      event "LegendVScrollShow": Value Change {
        w806 = T6 {"Left"=0, "Top"=0, "Right"=0, "Bottom"=0}  # input cluster
        n575 = event-data() -> ("NewVal"=w809:bool)  [unwired: 6 out]
        n576 = property on="Legend" class="MCListbox (strict)"("VScrollVis"=w809) -> ()  [unwired: 2 in, 2 out]
        n577 = control-ref of="PaneLegend"() -> (w807:refnum<vi>)
        n578 = property class="Pane"(reference=w807) -> ("Left"=w805:i32, "Top"=w802:i32, "Width"=w804:u32, "Height"=w801:u32)  [unwired: 1 in, 2 out]
        n579 = Add(x=w805, y=w804) -> (x+y=w803:u32)
        n580 = Add(x=w802, y=w801) -> (x+y=w800:u32)
        n581 = Bundle By Name(cluster=w806, "Left"=w805, "Top"=w802, "Right"=w803, "Bottom"=w800) -> (w799:T6)
        n582 = control-ref of="Legend"() -> (w808:refnum<vi>)
        n583 = local read "LegendVScrollShow"() -> (w798:bool)
        n584 = call "CRYLegend Resize in Graph Window.vi"("VScrollShow"=w798, "Pane Ref"=w807, "input cluster"=w799, "Legend"=w808) -> ()  [unwired: 8 out]
      }
      event "RemoveAll": Value Change {
        w818 = 0 ("Active X Scale")
        w816 = "" ("X Scale.Name Label.Text")
        n585 = event-data() -> ()  [unwired: 7 out]
        n586 = local write "TotalPlot"(u32 0 ("TotalPlot")) -> ()
        n587 = local write "OldRow"(-1 ("OldRow 2")) -> ()
        n588 = flat-sequence {
          frame #0 {
            n589 = control-ref of="This VI"() -> (w839:refnum<vi>)
            n590 = Build Array(-1 ("nData")) -> (w840:i32[])
            n591 = call "CRYSymbol Conversion.vi"("pGraph VI"=w839, "nDatas"=w840, "sActin"="LEGEND_REMOVE") -> ()  [unwired: 9 in]
          }
          frame #1 {
            n592 = control-ref of="Legend"() -> (w843:refnum<vi>)
            n593 = call "CRYData View Legend Item Delete.vi"("RowNumber"=-1, "Legend MultiListbox In"=w843) -> ()  [unwired: 10 out]
          }
        }
        n594 = flat-sequence {
          tunnel: w810 -> [w823]
          tunnel: [w823] -> w811
          tunnel: w811 -> [w831]
          frame #0 {
            n595 = local read "CursorShow"() -> (w822:bool)
            n596 = case shown="True" w822 {
              tunnel: w823 -> [_ w826]
              frame False {
              }
              frame True {
                n597 = local read "Graph Number"() -> (w824:i32)
                n598 = Format Into String("DA_CUR_HIDE" ("input 1"), "AAA" ("input 2"), w824, 0 ("input 3")) -> (resulting string=w828:string)  [unwired: 3 in, 1 out]
                n599 = Enqueue Element(queue=w826, element=w828) -> ()  [unwired: 1 in, 4 out]
              }
            }
          }
          frame #1 {
            n600 = local read "PreviewShow"() -> (w830:bool)
            n601 = case shown="True" w830 {
              tunnel: w831 -> [_ w834]
              frame False {
              }
              frame True {
                n602 = local read "Graph Number"() -> (w832:i32)
                n603 = Format Into String("DA_PRE_HIDE" ("input 1"), "AAA" ("input 2"), w832, 0 ("input 3")) -> (resulting string=w836:string)  [unwired: 3 in, 1 out]
                n604 = Enqueue Element(queue=w834, element=w836) -> ()  [unwired: 1 in, 4 out]
              }
            }
          }
        }
        n605 = local write "CursorEnabled"(FALSE ("CursorEnabled")) -> ()
        n606 = local write "XY Graph"(cluster{"XY Graph":cluster{dbl, dbl}[]}[] [] ("XY Graph")) -> ()
        n607 = property on="XY Graph" class="XYGraph (strict)"("ActXScl"=w818, "XScale.NameLbl.Text"=w816, "ActYScl"=w818, "YScale.NameLbl.Text"=w816, "ActYScl"=1 ("Active Y Scale"), "YScale.NameLbl.Text"=w816, "YScale.Visible"=FALSE ("Y Scale.Visible")) -> ()  [unwired: 2 in, 2 out]
        n608 = property on="PreviewGraph" class="XYGraph (strict)"("ActXScl"=0 ("Active X Scale"), "XScale.ScaleFit"=u8 2 ("X Scale.Scale Fit")) -> ()  [unwired: 2 in, 2 out]
      }
      event "RemoveSome": Value Change {
        n609 = event-data() -> ()  [unwired: 7 out]
        n610 = flat-sequence {
          tunnel: [w851] -> w845
          tunnel: [w856] -> w844
          tunnel: w845 -> [w879]
          tunnel: w844 -> [w878]
          frame #0 {
            n611 = control-ref of="Legend"() -> (w853:refnum<vi>)
            n612 = local read "SelectedRow"() -> (w852:i32[])
            n613 = call "CRYGet Phase Index.vi"("SelectedRow"=w852, "Legend Ref"=w853) -> ("CurveLibIndex"=w847:i32[], "LegendIndex"=w851:i32[])  [unwired: 8 in]
            n614 = control-ref of="Legend"() -> (w849:refnum<vi>)
            n615 = for {
              tunnel: w851 -> [w858] mode=indexing
              shift-right: [w859] -> w856
              shift-left: _ -> [w857]
              n616 = local read "TotalPlot"() -> (w863:u32)
              n617 = Decrement(x=w863) -> (x-1=w862:u32)
              n618 = Increment(x=w858) -> (x+1=w860:i32)
              n619 = Subtract(x=w862, y=w858) -> (x-y=w861:u32)
              n620 = for {
                N: w861 -> [_]
                tunnel: w860 -> [w870]
                shift-right: [w866] -> w859
                shift-left: w857 -> [w865]
                i -> [w869]
                n621 = Add(x=w870, y=w869) -> (x+y=w867:i32)
                n622 = Decrement(x=w867) -> (x-1=w868:i32)
                n623 = property on="XY Graph" class="XYGraph (strict)"(error in=w865, "Active Plot"=w867) -> (error out=w864:errorcluster, "Plot.Plot Color"=w877:u32, "Plot.Fill/Pt. Color"=w876:u32, "Plot.Fill To"=w875:i16, "Plot.Line Style"=w874:u8, "Plot.Line Width"=w873:u8, "Plot.Point Style"=w872:u8, "Plot.Plot Interpolation"=w871:u8)  [unwired: 1 in, 1 out]
                n624 = property on="XY Graph" class="XYGraph (strict)"(error in=w864, "Active Plot"=w868, "Plot.Plot Color"=w877, "Plot.Fill/Pt. Color"=w876, "Plot.Fill To"=w875, "Plot.Line Style"=w874, "Plot.Line Width"=w873, "Plot.Point Style"=w872, "Plot.Plot Interpolation"=w871) -> (error out=w866:errorcluster)  [unwired: 1 in, 1 out]
              }
              n625 = local write "TotalPlot"(w862) -> ()
            }
            n626 = local read "GraphType"() -> (w848:string)
            n627 = call "CRYData View Legend Manipulate.vi"("sAction"="GetGlobalNumbyLegNum", "nData"=w847, "sData"=w848, "Legend Ref"=w849) -> ("nData Out"=w846:i32[])  [unwired: 6 in, 1 out]
            n628 = control-ref of="This VI"() -> (w854:refnum<vi>)
            n629 = call "CRYSymbol Conversion.vi"("pGraph VI"=w854, "nDatas"=w846, "sActin"="LEGEND_REMOVE") -> ()  [unwired: 9 in]
          }
          frame #1 {
            n630 = case shown="No Error" w878 {
              frame No Error {
              }
              frame Error {
              }
            }
            n631 = for {
              tunnel: w879 -> [w880] mode=indexing
              n632 = control-ref of="Legend"() -> (w883:refnum<vi>)
              n633 = local read "XY Graph"() -> (w882:cluster{"XY Graph":cluster{dbl, dbl}[]}[])
              n634 = Delete From Array(array=w882, index=w880) -> (array with subset deleted=w881:cluster{"XY Graph":cluster{dbl, dbl}[]}[])  [unwired: 1 in, 1 out]
              n635 = call "CRYData View Legend Item Delete.vi"("RowNumber"=w880, "Legend MultiListbox In"=w883) -> ()  [unwired: 10 out]
              n636 = local write "XY Graph"(w881) -> ()
            }
          }
          frame #2 {
            n637 = local read "TotalPlot"() -> (w885:u32)
            n638 = case shown="1, Default" w885 {
              selector: w885 -> [_ w889]
              frame 0 {
                n639 = property on="RemoveAll" class="Bool (strict)"("Val(Sgnl)"=TRUE ("Value (Signaling)")) -> ()  [unwired: 2 in, 2 out]
              }
              frame 1, Default {
                n640 = for {
                  N: w889 -> [_]
                  tunnel: [w892] -> w887
                  i -> [w895]
                  n641 = property on="Legend" class="MCListbox (strict)"() -> ("ItemSyms"=w898:i32[])  [unwired: 2 in, 2 out]
                  n642 = Bundle By Name(cluster=T5 {"Row"=0, "Column"=0} ("Active Cell:Active Cell"), "Row"=w895, "Column"=1) -> (w899:T5)
                  n643 = Index Array(array=w898, index=w895) -> (element=w896:i32)
                  n644 = property on="Legend" class="MCListbox (strict)"("ActiveCell"=w899) -> ("CellBG"=w894:u32)  [unwired: 2 in, 2 out]
                  n645 = Equal?(x=w896, y=38) -> (x = y?=w893:bool)
                  n646 = property on="XY Graph" class="XYGraph (strict)"("Active Plot"=w895, "Plot.Plot Color"=w894, "Plot.Fill/Pt. Color"=w894, "Plot.Visible?"=w893) -> (error out=w892:errorcluster)  [unwired: 2 in, 1 out]
                }
                n647 = local read "PreviewShow"() -> (w888:bool)
                n648 = case shown="True" w888 {
                  frame False {
                  }
                  frame True {
                    n649 = control-ref of="This VI"() -> (w890:refnum<vi>)
                    n650 = call "CRYPlot XY Graph Preview.vi"("sOption"="Update", "Graph VI Ref"=w890) -> ()  [unwired: 10 in]
                  }
                }
                n651 = case shown="No Error" w887 {
                  frame No Error {
                  }
                  frame Error {
                  }
                }
              }
            }
            n652 = property on="AxisChange" class="Bool (strict)"("Val(Sgnl)"=TRUE ("Value (Signaling)")) -> ()  [unwired: 2 in, 2 out]
          }
        }
      }
      event "AxisChange": Value Change {
        w922 = enum16{"Curves", "Values", "Results", "WFM"}."Curves" ("Type In")
        n653 = event-data() -> ()  [unwired: 7 out]
        n654 = control-ref of="Legend"() -> (w927:refnum<vi>)
        n655 = call "CRYGet Graph Data in Graph.vi"("Graph Type"="XY", "Legend Refnum"=w927, "Type In"=w922) -> ("Rows"=w916:i32[])  [unwired: 4 in, 4 out]
        n656 = property on="Legend" class="MCListbox (strict)"() -> ("ItemSyms"=w928:i32[])  [unwired: 2 in, 2 out]
        n657 = call "CRYGet Legend Name.vi"("MCListbox Refnum"=w927) -> ("Names Out"=w921:string[])  [unwired: 10 in]
        n658 = local read "MagnitudeShow"() -> (w917:bool)
        n659 = local read "PhaseShow"() -> (w918:bool)
        n660 = control-ref of="This VI"() -> (w923:refnum<vi>)
        n661 = And(x=w917, y=w918) -> (x .and. y?=w910:bool)
        n662 = case shown="False" w910 {
          selector: w910 -> [w937 w938]
          tunnel: [w937 w938] -> w909
          frame False {
          }
          frame True {
            n663 = local write "AxisChangeOption"("AxisChange" ("AxisChange")) -> ()
          }
        }
        n664 = call "CRYMake Phase Index.vi"("Mag_Phase Flag"=w909, "Selected Rows In"=w916) -> ("Mag_Phase"=w913:bool[], "Selected Rows Out"=w915:i32[])  [unwired: 8 in]
        n665 = for {
          tunnel: w928 -> [w1004] mode=indexing
          shift-right: [w1003] -> w925
          shift-left: i32[] [] -> [w1002]
          tunnel: w915 -> [w1001] mode=indexing
          shift-right: [w998] -> w914
          shift-left: i32[] [] -> [w997]
          shift-right: [w995] -> w911
          shift-left: bool[] [] -> [w996]
          tunnel: w913 -> [w994] mode=indexing
          i -> [w999]
          n666 = Equal?(x=38, y=w1004) -> (x = y?=w1000:bool)
          n667 = case shown="True" w1000 {
            tunnel: [w1008 w1017] -> w1003
            tunnel: w1002 -> [w1008 w1016]
            tunnel: w1001 -> [_ w1015]
            tunnel: w999 -> [_ w1014]
            tunnel: [w1007 w1013] -> w998
            tunnel: w997 -> [w1007 w1012]
            tunnel: w996 -> [w1006 w1011]
            tunnel: [w1006 w1010] -> w995
            tunnel: w994 -> [_ w1009]
            frame False {
            }
            frame True {
              n668 = Insert Into Array(array=w1011, new element=w1009) -> (w1010:bool[])  [unwired: 1 in]
              n669 = Insert Into Array(array=w1012, new element=w1014) -> (w1013:i32[])  [unwired: 1 in]
              n670 = Insert Into Array(array=w1016, new element=w1015) -> (w1017:i32[])  [unwired: 1 in]
            }
          }
        }
        n671 = call "CRYGet Two Units Rows.vi"("Phase"=w911, "pGraph VI In"=w923, "Old Rows In"=w925, "Type"=w922) -> ("Unit2"=w930:string, "Unit1"=w926:string, "Two Units"=w931:i32)  [unwired: 1 in, 4 out]
        n672 = case shown="True" w910 {
          tunnel: w922 -> [_ w974]
          tunnel: w921 -> [w943 w973]
          tunnel: w914 -> [_ w972]
          tunnel: [w941 w971] -> w920
          tunnel: [w940 w970] -> w919
          tunnel: w917 -> [_ w969]
          frame True {
            n673 = for {
              tunnel: w943 -> [w947] mode=indexing
              tunnel: [w944] -> w940
              shift-right: [w945] -> w941
              shift-left: string[] [] -> [w946]
              n674 = Match Pattern(string=w947, regular expression=" \\[Phase\\]") -> (before substring=w954:string, after substring=w949:string, offset past match=w950:i32)  [unwired: 1 in, 1 out]
              n675 = Empty String/Path?(string/path=w949) -> (empty?=w952:bool)
              n676 = Greater Than 0?(x=w950) -> (x > 0?=w953:bool)
              n677 = And(x=w952, y=w953) -> (x .and. y?=w951:bool)
              n678 = case shown="False" w951 {
                tunnel: [w956 w963] -> w945
                tunnel: [w959 w966] -> w944
                tunnel: w947 -> [w958 _]
                tunnel: w954 -> [_ w965]
                tunnel: w946 -> [w957 w964]
                frame False {
                  n679 = call "CRYGet Curve Library Data.vi"("Type"=enum16{"Curves", "Values", "Results", "WFM"}."Curves", "Data Name"=w958) -> ("Curve"=w960:T9)  [unwired: 4 out]
                  n680 = Unbundle By Name(w960) -> ("Y unit"=w955:string, "X unit"=w959:string)  [unwired: 1 out]
                  n681 = Insert Into Array(array=w957, new element=w955) -> (w956:string[])  [unwired: 1 in]
                }
                frame True {
                  n682 = call "CRYGet Curve Library Data.vi"("Type"=enum16{"Curves", "Values", "Results", "WFM"}."Curves", "Data Name"=w965) -> ("Curve"=w967:T9)  [unwired: 4 out]
                  n683 = Unbundle By Name(w967) -> ("Z unit"=w962:string, "X unit"=w966:string)  [unwired: 1 out]
                  n684 = Insert Into Array(array=w964, new element=w962) -> (w963:string[])  [unwired: 1 in]
                }
              }
            }
          }
          frame False {
            n685 = for {
              tunnel: w973 -> [w983]
              tunnel: w972 -> [w984] mode=indexing
              tunnel: [w980] -> w975 mode=indexing
              tunnel: [w979] -> w976 mode=indexing
              tunnel: [w978] -> w970
              tunnel: w974 -> [w977]
              n686 = Index Array(array=w983, index=w984) -> (element=w982:string)
              n687 = call "CRYGet Curve Library Data.vi"("Type"=w977, "Data Name"=w982) -> ("Curve"=w981:T9)  [unwired: 4 out]
              n688 = Unbundle By Name(w981) -> ("Y unit"=w980:string, "Z unit"=w979:string, "X unit"=w978:string)
            }
            n689 = Select(t=w975, s=w969, f=w976) -> (s? t:f=w971:string[])
          }
        }
        n690 = property on="XY Graph" class="XYGraph (strict)"("ActYScl"=0 ("Active Y Scale")) -> (error out=w903:errorcluster, "YScale.NameLbl.Text"=w906:string)  [unwired: 2 in, 1 out]
        n691 = flat-sequence {
          tunnel: w904 -> [w933]
          frame #0 {
            n692 = case shown="True" w933 {
              frame False {
              }
              frame True {
                n693 = control-ref of="XY Graph"() -> (w934:refnum<vi>)
                n694 = control-ref of="This VI"() -> (w935:refnum<vi>)
                n695 = call "CRYSet Graph Scale.vi"("pGraph In"=w934, "pGraph VI In"=w935) -> ()  [unwired: 8 in, 2 out]
              }
            }
          }
          frame #1 {
            n696 = property on="Repaint Watermark" class="DigNum (strict)"("Val(Sgnl)"=-1 ("Value (Signaling)")) -> ()  [unwired: 2 in, 2 out]
          }
        }
        n697 = case shown="0" w931 {
          tunnel: w926 -> [w1020 _ w1033]
          tunnel: w930 -> [w1022 _ _]
          tunnel: w919 -> [w1018 _ w1031]
          tunnel: w903 -> [_ _ _]
          frame 2, Default {
            n698 = property on="XY Graph" class="XYGraph (strict)"("ActXScl"=0 ("Active X Scale"), "XScale.NameLbl.Text"=w1018, "ActYScl"=0 ("Active Y Scale"), "YScale.NameLbl.Text"=w1020, "ActYScl"=1 ("Active Y Scale"), "YScale.Visible"=TRUE ("Y Scale.Visible"), "YScale.NameLbl.Text"=w1022) -> ()  [unwired: 2 in, 2 out]
          }
          frame 0 {
            w1028 = 0 ("Active X Scale")
            w1026 = "" ("X Scale.Name Label.Text")
            n699 = property on="XY Graph" class="XYGraph (strict)"("ActXScl"=w1028, "XScale.NameLbl.Text"=w1026, "ActYScl"=w1028, "YScale.NameLbl.Text"=w1026, "ActYScl"=1 ("Active Y Scale"), "YScale.NameLbl.Text"=w1026, "YScale.Visible"=FALSE ("Y Scale.Visible")) -> ()  [unwired: 2 in, 2 out]
          }
          frame 1 {
            n700 = property on="XY Graph" class="XYGraph (strict)"("ActXScl"=0 ("Active X Scale"), "XScale.NameLbl.Text"=w1031, "ActYScl"=0 ("Active Y Scale"), "YScale.NameLbl.Text"=w1033, "ActYScl"=1 ("Active Y Scale"), "YScale.Visible"=FALSE ("Y Scale.Visible")) -> ()  [unwired: 2 in, 2 out]
          }
        }
        n701 = for {
          tunnel: w914 -> [w993] mode=indexing
          tunnel: w920 -> [w991] mode=indexing
          tunnel: w926 -> [w992]
          shift-right: [w986] -> w902
          shift-left: _ -> [w985]
          n702 = Equal?(x=w992, y=w991) -> (x = y?=w990:bool)
          n703 = Select(t=u32 0 ("Plot.Y Scale Index"), s=w990, f=u32 1 ("Plot.Y Scale Index")) -> (s? t:f=w987:u32)
          n704 = property on="XY Graph" class="XYGraph (strict)"(error in=w985, "Active Plot"=w993, "Plot.YScaleIdx"=w987) -> (error out=w986:errorcluster)  [unwired: 1 in, 1 out]
        }
        n705 = property on="XY Graph" class="XYGraph (strict)"(error in=w902, "ActYScl"=0 ("Active Y Scale")) -> ("YScale.NameLbl.Text"=w905:string)  [unwired: 1 in, 2 out]
        n706 = Not Equal?(x=w906, y=w905) -> (x != y?=w904:bool)
        n707 = case shown="No Error" w902 {
          frame No Error {
          }
          frame Error {
          }
        }
      }
      event "ColorBox": Value Change {
        # "Graph Color Changing"
        n708 = event-data() -> ("NewVal"=w1037:u32)  [unwired: 6 out]
        n709 = local read "OldRow"() -> (w1038:i32)
        n710 = local read "Event Name"() -> (w1035:string)
        n711 = flat-sequence {
          tunnel: [w1048] -> w1039
          tunnel: w1037 -> [w1048]
          tunnel: w1038 -> [w1047]
          tunnel: w1039 -> [w1049]
          frame #0 {
            n712 = To Unsigned Long Integer(number=w1047) -> (unsigned 32bit integer=w1046:u32)
            n713 = property on="XY Graph" class="XYGraph (strict)"("Active Plot"=w1046) -> (error out=w1045:errorcluster)  [unwired: 2 in, 1 out]
            n714 = property on="Legend" class="MCListbox (strict)"("CellBG"=w1048) -> ()  [unwired: 2 in, 2 out]
            n715 = case shown="No Error" w1045 {
              frame No Error {
              }
              frame Error {
              }
            }
          }
          frame #1 {
            n716 = property on="XY Graph" class="XYGraph (strict)"("Plot.Plot Color"=w1049) -> ()  [unwired: 2 in, 2 out]
            n717 = property on="ColorBox" class="ColBox"("Visible"=FALSE) -> ()  [unwired: 2 in, 2 out]
          }
        }
        n718 = call "CRYPreUpdate Sequence.vi"("EventName"="CurLibUpdate") -> ()  [unwired: 15 in]
        n719 = case shown="Default" w1035 {
          tunnel: w1038 -> [_ w1043]
          tunnel: w1037 -> [_ w1042]
          frame "ViewReport" {
          }
          frame Default {
            n720 = control-ref of="Legend"() -> (w1041:refnum<vi>)
            n721 = call "CRYSet Plot Settings.vi"("sAction"="Color", "Color"=w1042, "Row"=w1043, "Legend Refnum"=w1041, "Type"=enum16{"Curves", "Values", "Results", "WFM"}."Curves") -> ()  [unwired: 2 in, 5 out]
          }
        }
      }
      event "ColorBox": Mouse Down {
        n722 = event-data() -> ()  [unwired: 9 out]
        n723 = local read "OldRow"() -> (w1054:i32)
        n724 = Bundle By Name(cluster=T5 {"Row"=0, "Column"=0} ("Active Cell:Active Cell"), "Row"=w1054, "Column"=1) -> (w1051:T5)
        n725 = property on="Legend" class="MCListbox (strict)"("ActiveCell"=w1051) -> ()  [unwired: 2 in, 2 out]
      }
      event "XY Graph": Drag Enter {
        n726 = event-data() -> ("Available Data Names"=w1055:string[])  [unwired: 1 out]
        n727 = disable-structure shown="Disabled" {
          disable-tunnel: [w1058 TRUE] -> w1056
          disable-tunnel: w1055 -> [w1057 _]
          frame Disabled {
            n728 = Search 1D Array(1D array=w1057, element="CRY_GRAPH_DATA") -> (index of element=w1060:i32)  [unwired: 1 out]
            n729 = Not Equal?(x=w1060, y=-1) -> (x != y?=w1058:bool)
          }
          frame Enabled {
          }
        }
        n730 = event-data("Accepted?"=w1056) -> ()  [unwired: 1 in, 1 out]
      }
      event "XY Graph": Drop {
        n731 = event-data() -> ()  [unwired: 2 out]
        n732 = local read "Event Name"() -> (w1063:string)
        n733 = local read "TotalPlot"() -> (w1068:u32)
        n734 = control-ref of="This VI"() -> (w1064:refnum<vi>)
        n735 = call "CRYDrop Data in Same Graph.vi"("pGraph VI"=w1064, "Queue"=w1065, "Total Plot In"=w1068, "sAction"=w1063) -> ("Accepted?"=w1066:bool, "Total Plot Out"=w1067:u32)  [unwired: 3 in, 3 out]
        n736 = local write "TotalPlot"(w1067) -> ()
        n737 = event-data("Accepted?"=w1066) -> ()  [unwired: 1 in, 1 out]
      }
      event "XY Graph": Cursor Grab {
        n738 = event-data() -> ("CursIdx"=w1069:i32)  [unwired: 1 out]
        n739 = flat-sequence {
          tunnel: w1069 -> [w1070]
          frame #0 {
            n740 = Equal To 0?(x=w1070) -> (x = 0?=w1071:bool)
            n741 = local write "NewCursIdx"(w1070) -> ()
            n742 = Select(t=u32 1 ("OldCursIdx"), s=w1071, f=u32 0 ("OldCursIdx")) -> (s? t:f=w1074:u32)
            n743 = local write "OldCursIdx"(w1074) -> ()
          }
          frame #1 {
            n744 = property on="CursorColor" class="Bool (strict)"("Val(Sgnl)"=TRUE ("Value (Signaling)")) -> ()  [unwired: 2 in, 2 out]
          }
        }
      }
      event "XY Graph": Cursor Move {
        n745 = event-data() -> ()  [unwired: 10 out]
        n746 = property on="CursorPlot" class="Bool (strict)"("Val(Sgnl)"=TRUE ("Value (Signaling)")) -> ()  [unwired: 2 in, 2 out]
      }
      event "ReportDrop": Value Change {
        n747 = event-data() -> ()  [unwired: 7 out]
        n748 = local read "Event Name"() -> (w1077:string)
        n749 = local read "TotalPlot"() -> (w1081:u32)
        n750 = control-ref of="This VI"() -> (w1079:refnum<vi>)
        n751 = call "CRYDrop Data in Same Graph.vi"("pGraph VI"=w1079, "Queue"=w1078, "Total Plot In"=w1081, "sAction"=w1077) -> ("Total Plot Out"=w1080:u32)  [unwired: 3 in, 4 out]
        n752 = local write "TotalPlot"(w1080) -> ()
      }
      event "XY Graph": Scale Range Change {
        n753 = event-data() -> ("Kind"=w1083:enum16{"X-Scale", "Y-Scale", "Z-Scale"})  [unwired: 8 out]
        n754 = local read "PreviewShow"() -> (w1082:bool)
        n755 = case shown="\"Y-Scale\"" w1083 {
          frame "X-Scale", Default {
            w1085 = u8 0 ("X Scale.Scale Fit")
            n756 = property on="XY Graph" class="XYGraph (strict)"("XScale.ScaleFit"=w1085) -> ()  [unwired: 2 in, 2 out]
            n757 = property on="PreviewGraph" class="XYGraph (strict)"("XScale.ScaleFit"=w1085) -> ()  [unwired: 2 in, 2 out]
          }
          frame "Y-Scale" {
            n758 = property on="Repaint Watermark" class="DigNum (strict)"("Val(Sgnl)"=-1 ("y")) -> ()  [unwired: 2 in, 2 out]
            n759 = property on="XY Graph" class="XYGraph (strict)"("YScale.ScaleFit"=u8 0 ("Y Scale.Scale Fit")) -> ()  [unwired: 2 in, 2 out]
          }
        }
        n760 = case shown="True" w1082 {
          frame False {
          }
          frame True {
            n761 = property on="ScaleRange" class="Bool (strict)"("Val(Sgnl)"=TRUE ("Value (Signaling)")) -> ()  [unwired: 2 in, 2 out]
          }
        }
      }
      event "ScaleRange": Value Change {
        n762 = event-data() -> ()  [unwired: 7 out]
        n763 = disable-structure shown="Disabled" {
          frame Disabled {
            n764 = property on="XY Graph" class="XYGraph (strict)"() -> ("XScale.Maximum"=w1116:dbl, "XScale.Minimum"=w1117:dbl)  [unwired: 2 in, 2 out]
            n765 = property on="PreviewGraph" class="XYGraph (strict)"() -> ("XScale.Maximum"=w1101:dbl, "XScale.Minimum"=w1095:dbl)  [unwired: 2 in, 2 out]
            n766 = Greater?(x=w1095, y=w1117) -> (0:w1118:bool)
            n767 = Less?(x=w1101, y=w1116) -> (x < y?=w1115:bool)
            n768 = Subtract(x=w1101, y=w1095) -> (x-y=w1100:dbl)
            n769 = Select(t=w1101, s=w1115, f=w1116) -> (s? t:f=w1096:dbl)
            n770 = Select(t=w1095, s=w1118, f=w1117) -> (s? t:f=w1097:dbl)
            n771 = Subtract(x=w1097, y=w1095) -> (x-y=w1094:dbl)
            n772 = Subtract(x=w1096, y=w1095) -> (x-y=w1093:dbl)
            n773 = property on="PreviewGraph" class="XYGraph (strict)"("Active Cursor"=u32 0, "Cursor.Cursor X"=w1097, "Active Cursor"=u32 1, "Cursor.Cursor X"=w1096) -> (error out=w1114:errorcluster)  [unwired: 2 in, 1 out]
            n774 = Divide(x=w1094, y=w1100) -> (x/y=w1098:dbl)
            n775 = Divide(x=w1093, y=w1100) -> (x/y=w1099:dbl)
            n776 = property on="Scrollbar" class="Scroll (strict)"() -> ("DocMax"=w1107:dbl, "PageSize"=w1089:dbl)  [unwired: 2 in, 2 out]
            n777 = Subtract(x=w1098, y=w1099) -> (x-y=w1105:dbl)
            n778 = flat-sequence {
              tunnel: w1114 -> [_]
              frame #0 {
                n779 = control-ref of="This VI"() -> (w1120:refnum<vi>)
                n780 = call "CRYPlot XY Graph Preview.vi"("sOption"="Move", "Graph VI Ref"=w1120) -> ()  [unwired: 10 in]
              }
            }
            n781 = Divide(x=w1089, y=w1105) -> (x/y=w1104:dbl)
            n782 = local read "ScaleMax"() -> (w1103:dbl)
            n783 = local read "ScaleMin"() -> (w1102:dbl)
            n784 = Add(x=w1107, y=w1104) -> (x+y=w1106:dbl)
            n785 = property on="Scrollbar" class="Scroll (strict)"("DocMin"=w1106) -> ("DocMax"=w1091:dbl, "DocMin"=w1090:dbl)  [unwired: 2 in, 2 out]
            n786 = Subtract(x=w1103, y=w1102) -> (x-y=w1092:dbl)
            n787 = Subtract(x=w1098, y=w1102) -> (x-y=w1108:dbl)
            n788 = Subtract(x=w1091, y=w1090) -> (x-y=w1109:dbl)
            n789 = Multiply(x=w1108, y=w1109) -> (x*y=w1110:dbl)
            n790 = Divide(x=w1110, y=w1092) -> (x/y=w1111:dbl)
            n791 = Add(x=w1111, y=w1090) -> (x+y=w1088:dbl)
            n792 = property on="Scrollbar" class="Scroll (strict)"("Value"=w1088) -> ()  [unwired: 2 in, 2 out]
          }
          frame Enabled {
          }
        }
      }
      event "Repaint Watermark": Value Change {
        # "Repaint Watermark: 0-none, 1-Unit 1, 2-Unit 1 & 2, -1: surely replot"
        n793 = event-data() -> ("OldVal"=w1126:i32, "NewVal"=w1122:i32)  [unwired: 5 out]
        n794 = Equal?(x=-1 ("y"), y=w1122) -> (x = y?=w1123:bool)
        n795 = case shown="False" w1123 {
          tunnel: w1126 -> [w1129 w1144]
          tunnel: [w1128 "Replot" ("PropertyTab")] -> w1125
          tunnel: w1122 -> [w1127 _]
          tunnel: [w1127 w1144] -> w1121
          frame False {
            n796 = Not Equal?(x=w1129, y=w1127) -> (x != y?=w1130:bool)
            n797 = case shown="True" w1130 {
              tunnel: w1129 -> [_ w1137]
              tunnel: w1127 -> [_ w1136]
              tunnel: [_ w1131] -> w1128
              frame False {
              }
              frame True {
                n798 = Equal To 0?(x=w1137) -> (x = 0?=w1141:bool)
                n799 = Equal?(x=w1136, y=1) -> (x = y?=w1142:bool)
                n800 = Equal?(x=w1137, y=1) -> (x = y?=w1135:bool)
                n801 = Equal To 0?(x=w1136) -> (x = 0?=w1134:bool)
                n802 = And(x=w1135, y=w1134) -> (x .and. y?=w1133:bool)
                n803 = And(x=w1141, y=w1142) -> (x .and. y?=w1139:bool)
                n804 = Or(x=w1139, y=w1133) -> (x .or. y?=w1132:bool)
                n805 = case shown="False" w1132 {
                  tunnel: ["Replot" ("PropertyTab") _] -> w1131
                  frame False {
                  }
                  frame True {
                  }
                }
              }
            }
          }
          frame True {
          }
        }
        n806 = local write "Repaint Watermark"(w1121) -> ()
        n807 = case shown="\"Replot\"" w1125 {
          frame Default {
          }
          frame "Replot" {
            n808 = local read "Event Name"() -> (w1146:string)
            n809 = control-ref of="XY Graph"() -> (w1147:refnum<vi>)
            n810 = call "CRYPaint WaterMark.vi"("Type"=w1146, "Graph Ref"=w1147) -> ()  [unwired: 10 in]
          }
        }
      }
      event "PreviewGraph": Cursor Move {
        n811 = event-data() -> ("CursIdx"=w1148:i32, "CursLoc"=w1149:cluster{"X":dbl, "Y":dbl})  [unwired: 1 out]
        n812 = disable-structure shown="Disabled" {
          disable-tunnel: w1149 -> [w1151 _]
          disable-tunnel: w1148 -> [w1150 _]
          frame Disabled {
            n813 = property on="PreviewGraph" class="XYGraph (strict)"("ActXScl"=0 ("Active X Scale")) -> ("XScale.Maximum"=w1160:dbl, "XScale.Minimum"=w1159:dbl)  [unwired: 2 in, 2 out]
            n814 = property on="XY Graph" class="XYGraph (strict)"("ActXScl"=0 ("Active X Scale"), "XScale.ScaleFit"=u8 0 ("X Scale.Scale Fit")) -> ()  [unwired: 2 in, 2 out]
            n815 = Unbundle By Name(w1151) -> ("X"=w1152:dbl)
            n816 = Less Or Equal?(x=w1152, y=w1159) -> (x <= y?=w1156:bool)
            n817 = Greater Or Equal?(x=w1152, y=w1160) -> (x >= y?=w1155:bool)
            n818 = Or(x=w1156, y=w1155) -> (x .or. y?=w1157:bool)
            n819 = case shown="True" w1157 {
              tunnel: w1156 -> [_ w1208]
              tunnel: w1150 -> [_ w1203]
              frame False {
                n820 = property on="PreviewGraph" class="XYGraph (strict)"("Active Cursor"=u32 0, "Active Cursor"=u32 1) -> ("Cursor.Cursor X"=w1181:dbl, "Cursor.Cursor X"=w1182:dbl)  [unwired: 2 in, 2 out]
                n821 = property on="PreviewGraph" class="XYGraph (strict)"("ActXScl"=0 ("Active X Scale")) -> ("XScale.Maximum"=w1175:dbl, "XScale.Minimum"=w1174:dbl)  [unwired: 2 in, 2 out]
                n822 = control-ref of="This VI"() -> (w1164:refnum<vi>)
                n823 = property on="XY Graph" class="XYGraph (strict)"("ActXScl"=0 ("Active X Scale"), "XScale.ScaleFit"=u8 0 ("X Scale.Scale Fit")) -> (error out=w1165:errorcluster)  [unwired: 2 in, 1 out]
                n824 = Greater?(x=w1181, y=w1182) -> (0:w1180:bool)
                n825 = case shown="True" w1180 {
                  tunnel: w1181 -> [w1200 w1202]
                  tunnel: w1182 -> [w1199 w1201]
                  tunnel: [w1200 w1201] -> w1168
                  tunnel: [w1199 w1202] -> w1176
                  frame False {
                  }
                  frame True {
                  }
                }
                n826 = call "CRYPlot XY Graph Preview.vi"("sOption"="Move", "Graph VI Ref"=w1164) -> ()  [unwired: 10 in]
                n827 = Subtract(x=w1175, y=w1174) -> (x-y=w1170:dbl)
                n828 = property on="XY Graph" class="XYGraph (strict)"(error in=w1165, "XScale.Minimum"=w1168, "XScale.Maximum"=w1176) -> ()  [unwired: 1 in, 2 out]
                n829 = Subtract(x=w1168, y=w1174) -> (x-y=w1173:dbl)
                n830 = Subtract(x=w1176, y=w1174) -> (x-y=w1171:dbl)
                n831 = Divide(x=w1173, y=w1170) -> (x/y=w1172:dbl)
                n832 = Divide(x=w1171, y=w1170) -> (x/y=w1169:dbl)
                n833 = Subtract(x=w1172, y=w1169) -> (x-y=w1161:dbl)
                n834 = Equal To 0?(x=w1161) -> (x = 0?=w1162:bool)
                n835 = case shown="False" w1162 {
                  tunnel: w1161 -> [w1187 _]
                  tunnel: w1172 -> [w1183 _]
                  frame False {
                    n836 = property on="Scrollbar" class="Scroll (strict)"() -> ("DocMax"=w1189:dbl, "PageSize"=w1196:dbl)  [unwired: 2 in, 2 out]
                    n837 = Divide(x=w1196, y=w1187) -> (x/y=w1186:dbl)
                    n838 = local read "ScaleMax"() -> (w1185:dbl)
                    n839 = local read "ScaleMin"() -> (w1184:dbl)
                    n840 = Add(x=w1189, y=w1186) -> (x+y=w1188:dbl)
                    n841 = property on="Scrollbar" class="Scroll (strict)"("DocMin"=w1188) -> ("DocMax"=w1198:dbl, "DocMin"=w1197:dbl)  [unwired: 2 in, 2 out]
                    n842 = Subtract(x=w1185, y=w1184) -> (x-y=w1193:dbl)
                    n843 = Subtract(x=w1183, y=w1184) -> (x-y=w1190:dbl)
                    n844 = Subtract(x=w1198, y=w1197) -> (x-y=w1191:dbl)
                    n845 = Multiply(x=w1190, y=w1191) -> (x*y=w1192:dbl)
                    n846 = Divide(x=w1192, y=w1193) -> (x/y=w1194:dbl)
                    n847 = Add(x=w1194, y=w1197) -> (x+y=w1195:dbl)
                    n848 = property on="Scrollbar" class="Scroll (strict)"("Value"=w1195) -> ()  [unwired: 2 in, 2 out]
                  }
                  frame True {
                  }
                }
              }
              frame True {
                n849 = property on="PreviewGraph" class="XYGraph (strict)"("ActXScl"=0 ("Active X Scale")) -> ("XScale.Maximum"=w1206:dbl, "XScale.Minimum"=w1207:dbl)  [unwired: 2 in, 2 out]
                n850 = Subtract(x=w1206, y=w1207) -> (x-y=w1209:dbl)
                n851 = case shown="False" w1208 {
                  tunnel: w1207 -> [w1216 _]
                  tunnel: w1206 -> [_ w1219]
                  tunnel: [w1215 w1218] -> w1205
                  tunnel: w1203 -> [w1214 w1217]
                  frame True {
                    n852 = property on="PreviewGraph" class="XYGraph (strict)"("Active Cursor"=w1214, "Cursor.Cursor X"=w1216) -> (error out=w1215:errorcluster)  [unwired: 2 in, 1 out]
                  }
                  frame False {
                    n853 = property on="PreviewGraph" class="XYGraph (strict)"("Active Cursor"=w1217, "Cursor.Cursor X"=w1219) -> (error out=w1218:errorcluster)  [unwired: 2 in, 1 out]
                  }
                }
                n854 = flat-sequence {
                  tunnel: w1207 -> [w1226]
                  tunnel: w1209 -> [w1223]
                  tunnel: w1204 -> [w1220]
                  frame #0 {
                    n855 = property on="PreviewGraph" class="XYGraph (strict)"(error in=w1220, "Active Cursor"=u32 0, "Active Cursor"=u32 1) -> ("Cursor.Cursor X"=w1230:dbl, "Cursor.Cursor X"=w1229:dbl)  [unwired: 1 in, 2 out]
                    n856 = Greater?(x=w1230, y=w1229) -> (0:w1246:bool)
                    n857 = case shown="True" w1246 {
                      tunnel: w1230 -> [w1250 w1252]
                      tunnel: w1229 -> [w1249 w1251]
                      tunnel: [w1250 w1251] -> w1228
                      tunnel: [w1249 w1252] -> w1227
                      frame False {
                      }
                      frame True {
                      }
                    }
                    n858 = Subtract(x=w1228, y=w1226) -> (x-y=w1225:dbl)
                    n859 = Subtract(x=w1227, y=w1226) -> (x-y=w1222:dbl)
                    n860 = Divide(x=w1225, y=w1223) -> (x/y=w1224:dbl)
                    n861 = Divide(x=w1222, y=w1223) -> (x/y=w1221:dbl)
                    n862 = property on="XY Graph" class="XYGraph (strict)"("XScale.Minimum"=w1228, "XScale.Maximum"=w1227) -> ()  [unwired: 2 in, 2 out]
                    n863 = property on="Scrollbar" class="Scroll (strict)"() -> ("DocMax"=w1240:dbl, "PageSize"=w1233:dbl)  [unwired: 2 in, 2 out]
                    n864 = Subtract(x=w1224, y=w1221) -> (x-y=w1242:dbl)
                    n865 = local read "ScaleMax"() -> (w1244:dbl)
                    n866 = local read "ScaleMin"() -> (w1245:dbl)
                    n867 = Divide(x=w1233, y=w1242) -> (x/y=w1243:dbl)
                    n868 = Add(x=w1240, y=w1243) -> (x+y=w1241:dbl)
                    n869 = property on="Scrollbar" class="Scroll (strict)"("DocMin"=w1241) -> ("DocMax"=w1231:dbl, "DocMin"=w1232:dbl)  [unwired: 2 in, 2 out]
                    n870 = Subtract(x=w1244, y=w1245) -> (x-y=w1236:dbl)
                    n871 = Subtract(x=w1224, y=w1245) -> (x-y=w1239:dbl)
                    n872 = Subtract(x=w1231, y=w1232) -> (x-y=w1238:dbl)
                    n873 = Multiply(x=w1239, y=w1238) -> (x*y=w1237:dbl)
                    n874 = Divide(x=w1237, y=w1236) -> (x/y=w1235:dbl)
                    n875 = Add(x=w1235, y=w1232) -> (x+y=w1234:dbl)
                    n876 = property on="Scrollbar" class="Scroll (strict)"("Value"=w1234) -> ()  [unwired: 2 in, 2 out]
                  }
                }
                n877 = flat-sequence {
                  tunnel: w1205 -> [w1211]
                  tunnel: [w1211] -> w1204
                  frame #0 {
                    n878 = control-ref of="This VI"() -> (w1213:refnum<vi>)
                    n879 = call "CRYPlot XY Graph Preview.vi"("sOption"="Move", "Graph VI Ref"=w1213) -> ()  [unwired: 10 in]
                  }
                }
              }
            }
          }
          frame Enabled {
          }
        }
      }
      event "PreviewGraph": Mouse Down {
        n880 = event-data() -> ("Button"=w1253:u16, "Coords"=w1254:T1)  [unwired: 1 out]
        n881 = disable-structure shown="Disabled" {
          disable-tunnel: w1254 -> [w1256 _]
          disable-tunnel: w1253 -> [w1255 _]
          frame Disabled {
            n882 = case shown="Default" w1255 {
              tunnel: w1256 -> [w1268 w1394]
              frame Default {
                n883 = property on="PreviewGraph" class="XYGraph (strict)"() -> ("Plot Bounds"=w1269:T6, "Width"=w1267:u32)  [unwired: 2 in, 2 out]
                n884 = Unbundle By Name(w1268) -> ("Horizontal"=w1263:i32)
                n885 = property on="PreviewGraph" class="XYGraph (strict)"("ActXScl"=0 ("Active X Scale"), "XScale.ScaleFit"=u8 0 ("X Scale.Scale Fit")) -> ()  [unwired: 2 in, 2 out]
                n886 = To Long Integer(number=w1267) -> (32bit integer=w1260:i32)
                n887 = Unbundle By Name(w1269) -> ("Left"=w1266:i16)
                n888 = To Long Integer(number=w1266) -> (32bit integer=w1261:i32)
                n889 = Add(x=w1261, y=w1260) -> (x+y=w1262:i32)
                n890 = Less?(x=w1263, y=w1261) -> (x < y?=w1257:bool)
                n891 = Greater?(x=w1263, y=w1262) -> (0:w1264:bool)
                n892 = Or(x=w1257, y=w1264) -> (x .or. y?=w1265:bool)
                n893 = case shown="False" w1265 {
                  tunnel: w1261 -> [w1274 _]
                  tunnel: w1260 -> [w1273 _]
                  tunnel: w1263 -> [w1272 _]
                  tunnel: w1257 -> [_ w1348]
                  frame False {
                    n894 = property on="PreviewGraph" class="XYGraph (strict)"("ActXScl"=0 ("Active X Scale")) -> ("XScale.Maximum"=w1284:dbl, "XScale.Minimum"=w1280:dbl)  [unwired: 2 in, 2 out]
                    n895 = property on="PreviewGraph" class="XYGraph (strict)"("Active Cursor"=u32 0, "Active Cursor"=u32 1) -> ("Cursor.Cursor X"=w1271:dbl, "Cursor.Cursor X"=w1270:dbl)  [unwired: 2 in, 2 out]
                    n896 = Subtract(x=w1272, y=w1274) -> (x-y=w1287:i32)
                    n897 = Divide(x=w1287, y=w1273) -> (x/y=w1283:dbl)
                    n898 = Subtract(x=w1284, y=w1280) -> (x-y=w1279:dbl)
                    n899 = Less Or Equal?(x=w1271, y=w1270) -> (x <= y?=w1291:bool)
                    n900 = Multiply(x=w1283, y=w1279) -> (x*y=w1282:dbl)
                    n901 = Subtract(x=w1271, y=w1270) -> (x-y=w1278:dbl)
                    n902 = flat-sequence {
                      tunnel: w1292 -> [_]
                      tunnel: w1280 -> [w1298]
                      tunnel: w1279 -> [w1295]
                      frame #0 {
                        n903 = property on="PreviewGraph" class="XYGraph (strict)"("Active Cursor"=u32 0, "Active Cursor"=u32 1) -> ("Cursor.Cursor X"=w1302:dbl, "Cursor.Cursor X"=w1301:dbl)  [unwired: 2 in, 2 out]
                        n904 = Greater?(x=w1302, y=w1301) -> (0:w1318:bool)
                        n905 = case shown="True" w1318 {
                          tunnel: w1302 -> [w1322 w1324]
                          tunnel: w1301 -> [w1321 w1323]
                          tunnel: [w1322 w1323] -> w1300
                          tunnel: [w1321 w1324] -> w1299
                          frame False {
                          }
                          frame True {
                          }
                        }
                        n906 = Subtract(x=w1300, y=w1298) -> (x-y=w1297:dbl)
                        n907 = Subtract(x=w1299, y=w1298) -> (x-y=w1294:dbl)
                        n908 = Divide(x=w1297, y=w1295) -> (x/y=w1296:dbl)
                        n909 = Divide(x=w1294, y=w1295) -> (x/y=w1293:dbl)
                        n910 = property on="XY Graph" class="XYGraph (strict)"("XScale.Minimum"=w1300, "XScale.Maximum"=w1299) -> ()  [unwired: 2 in, 2 out]
                        n911 = property on="Scrollbar" class="Scroll (strict)"() -> ("DocMax"=w1312:dbl, "PageSize"=w1305:dbl)  [unwired: 2 in, 2 out]
                        n912 = Subtract(x=w1296, y=w1293) -> (x-y=w1314:dbl)
                        n913 = local read "ScaleMax"() -> (w1316:dbl)
                        n914 = local read "ScaleMin"() -> (w1317:dbl)
                        n915 = Divide(x=w1305, y=w1314) -> (x/y=w1315:dbl)
                        n916 = Add(x=w1312, y=w1315) -> (x+y=w1313:dbl)
                        n917 = property on="Scrollbar" class="Scroll (strict)"("DocMin"=w1313) -> ("DocMax"=w1303:dbl, "DocMin"=w1304:dbl)  [unwired: 2 in, 2 out]
                        n918 = Subtract(x=w1316, y=w1317) -> (x-y=w1308:dbl)
                        n919 = Subtract(x=w1296, y=w1317) -> (x-y=w1311:dbl)
                        n920 = Subtract(x=w1303, y=w1304) -> (x-y=w1310:dbl)
                        n921 = Multiply(x=w1311, y=w1310) -> (x*y=w1309:dbl)
                        n922 = Divide(x=w1309, y=w1308) -> (x/y=w1307:dbl)
                        n923 = Add(x=w1307, y=w1304) -> (x+y=w1306:dbl)
                        n924 = property on="Scrollbar" class="Scroll (strict)"("Value"=w1306) -> ()  [unwired: 2 in, 2 out]
                      }
                    }
                    n925 = Absolute Value(x=w1278) -> (abs(x)=w1277:dbl)
                    n926 = Add(x=w1282, y=w1280) -> (x+y=w1281:dbl)
                    n927 = Divide(x=w1277, y=2.0) -> (x/y=w1275:dbl)
                    n928 = case shown="True" w1291 {
                      tunnel: [w1329 w1337] -> w1289
                      tunnel: w1281 -> [w1325 w1334]
                      tunnel: w1271 -> [w1328 _]
                      tunnel: w1270 -> [_ w1333]
                      tunnel: w1275 -> [w1327 w1336]
                      frame True {
                        n929 = Add(x=w1328, y=w1327) -> (x+y=w1326:dbl)
                        n930 = Greater?(x=w1326, y=w1325) -> (0:w1332:bool)
                        n931 = Select(t=u32 0 ("Active Cursor"), s=w1332, f=u32 1) -> (s? t:f=w1329:u32)
                      }
                      frame False {
                        n932 = Add(x=w1333, y=w1336) -> (x+y=w1335:dbl)
                        n933 = Greater?(x=w1335, y=w1334) -> (0:w1340:bool)
                        n934 = Select(t=u32 1 ("Active Cursor"), s=w1340, f=u32 0) -> (s? t:f=w1337:u32)
                      }
                    }
                    n935 = property on="PreviewGraph" class="XYGraph (strict)"("Active Cursor"=w1289, "Cursor.Cursor X"=w1281) -> (error out=w1288:errorcluster)  [unwired: 2 in, 1 out]
                    n936 = flat-sequence {
                      tunnel: w1288 -> [w1343]
                      tunnel: [w1343] -> w1292
                      frame #0 {
                        n937 = control-ref of="This VI"() -> (w1342:refnum<vi>)
                        n938 = call "CRYPlot XY Graph Preview.vi"("sOption"="Move", "Graph VI Ref"=w1342) -> ()  [unwired: 10 in]
                      }
                    }
                  }
                  frame True {
                    n939 = property on="PreviewGraph" class="XYGraph (strict)"("ActXScl"=0 ("Active X Scale")) -> ("XScale.Maximum"=w1347:dbl, "XScale.Minimum"=w1346:dbl)  [unwired: 2 in, 2 out]
                    n940 = Subtract(x=w1347, y=w1346) -> (x-y=w1349:dbl)
                    n941 = case shown="False" w1348 {
                      tunnel: w1347 -> [_ w1356]
                      tunnel: w1346 -> [w1352 _]
                      tunnel: [w1351 w1355] -> w1345
                      frame True {
                        n942 = property on="PreviewGraph" class="XYGraph (strict)"("Active Cursor"=u32 0, "Cursor.Cursor X"=w1352, "Active Cursor"=u32 1, "Cursor.Cursor X"=w1352) -> (error out=w1351:errorcluster)  [unwired: 2 in, 1 out]
                      }
                      frame False {
                        n943 = property on="PreviewGraph" class="XYGraph (strict)"("Active Cursor"=u32 0, "Cursor.Cursor X"=w1356, "Active Cursor"=u32 1, "Cursor.Cursor X"=w1356) -> (error out=w1355:errorcluster)  [unwired: 2 in, 1 out]
                      }
                    }
                    n944 = flat-sequence {
                      tunnel: w1346 -> [w1364]
                      tunnel: w1349 -> [w1361]
                      tunnel: w1344 -> [_]
                      frame #0 {
                        n945 = property on="PreviewGraph" class="XYGraph (strict)"("Active Cursor"=u32 0, "Active Cursor"=u32 1) -> ("Cursor.Cursor X"=w1368:dbl, "Cursor.Cursor X"=w1367:dbl)  [unwired: 2 in, 2 out]
                        n946 = Greater?(x=w1368, y=w1367) -> (0:w1384:bool)
                        n947 = case shown="True" w1384 {
                          tunnel: w1368 -> [w1388 w1390]
                          tunnel: w1367 -> [w1387 w1389]
                          tunnel: [w1388 w1389] -> w1366
                          tunnel: [w1387 w1390] -> w1365
                          frame False {
                          }
                          frame True {
                          }
                        }
                        n948 = Subtract(x=w1366, y=w1364) -> (x-y=w1363:dbl)
                        n949 = Subtract(x=w1365, y=w1364) -> (x-y=w1360:dbl)
                        n950 = Divide(x=w1363, y=w1361) -> (x/y=w1362:dbl)
                        n951 = Divide(x=w1360, y=w1361) -> (x/y=w1359:dbl)
                        n952 = property on="XY Graph" class="XYGraph (strict)"("XScale.Minimum"=w1366, "XScale.Maximum"=w1365) -> ()  [unwired: 2 in, 2 out]
                        n953 = property on="Scrollbar" class="Scroll (strict)"() -> ("DocMax"=w1378:dbl, "PageSize"=w1371:dbl)  [unwired: 2 in, 2 out]
                        n954 = Subtract(x=w1362, y=w1359) -> (x-y=w1380:dbl)
                        n955 = local read "ScaleMax"() -> (w1382:dbl)
                        n956 = local read "ScaleMin"() -> (w1383:dbl)
                        n957 = Divide(x=w1371, y=w1380) -> (x/y=w1381:dbl)
                        n958 = Add(x=w1378, y=w1381) -> (x+y=w1379:dbl)
                        n959 = property on="Scrollbar" class="Scroll (strict)"("DocMin"=w1379) -> ("DocMax"=w1369:dbl, "DocMin"=w1370:dbl)  [unwired: 2 in, 2 out]
                        n960 = Subtract(x=w1382, y=w1383) -> (x-y=w1374:dbl)
                        n961 = Subtract(x=w1362, y=w1383) -> (x-y=w1377:dbl)
                        n962 = Subtract(x=w1369, y=w1370) -> (x-y=w1376:dbl)
                        n963 = Multiply(x=w1377, y=w1376) -> (x*y=w1375:dbl)
                        n964 = Divide(x=w1375, y=w1374) -> (x/y=w1373:dbl)
                        n965 = Add(x=w1373, y=w1370) -> (x+y=w1372:dbl)
                        n966 = property on="Scrollbar" class="Scroll (strict)"("Value"=w1372) -> ()  [unwired: 2 in, 2 out]
                      }
                    }
                    n967 = flat-sequence {
                      tunnel: w1345 -> [w1391]
                      tunnel: [w1391] -> w1344
                      frame #0 {
                        n968 = control-ref of="This VI"() -> (w1393:refnum<vi>)
                        n969 = call "CRYPlot XY Graph Preview.vi"("sOption"="Move", "Graph VI Ref"=w1393) -> ()  [unwired: 10 in]
                      }
                    }
                  }
                }
              }
              frame 2 {
                n970 = local write "PreviewCoords"(w1394) -> ()
              }
            }
          }
          frame Enabled {
          }
        }
      }
      event "PreviewShow": Value Change {
        n971 = event-data() -> ("NewVal"=w1395:bool)  [unwired: 6 out]
        n972 = disable-structure shown="Disabled" {
          disable-tunnel: w1395 -> [w1396 _]
          frame Disabled {
            n973 = flat-sequence {
              tunnel: w1396 -> [w1401]
              frame #0 {
                n974 = Select(t="DA_PRE_VIEW", s=w1401, f="DA_PRE_HIDE") -> (s? t:f=w1400:string)
                n975 = control-ref of="This VI"() -> (w1397:refnum<vi>)
                n976 = call "CRYPreview InsDel.vi"("Graph VI Ref"=w1397, "sAction"=w1400) -> ()  [unwired: 10 in]
              }
              frame #1 {
                n977 = property on="ToolbarUpdate" class="Bool (strict)"("Val(Sgnl)"=TRUE ("Value (Signaling)")) -> ()  [unwired: 2 in, 2 out]
              }
            }
          }
          frame Enabled {
          }
        }
      }
      event "PreviewGraph": Scale Range Change {
        n978 = event-data() -> ("NewRange"=w1403:T10)  [unwired: 8 out]
        n979 = disable-structure shown="Disabled" {
          disable-tunnel: w1403 -> [w1404 _]
          frame Disabled {
            n980 = local read "PreviewScaleMax"() -> (w1411:dbl)
            n981 = local read "PreviewScaleMin"() -> (w1410:dbl)
            n982 = Unbundle By Name(w1404) -> ("Minimum"=w1405:dbl, "Maximum"=w1406:dbl)
            n983 = Less?(x=w1405, y=w1410) -> (x < y?=w1407:bool)
            n984 = Greater?(x=w1406, y=w1411) -> (0:w1408:bool)
            n985 = Or(x=w1407, y=w1408) -> (x .or. y?=w1409:bool)
            n986 = case shown="True" w1409 {
              tunnel: w1410 -> [_ w1414]
              tunnel: w1411 -> [_ w1413]
              frame False {
              }
              frame True {
                n987 = property on="PreviewGraph" class="XYGraph (strict)"("ActXScl"=0 ("Active X Scale"), "XScale.Maximum"=w1413, "XScale.Minimum"=w1414) -> (error out=w1412:errorcluster)  [unwired: 2 in, 1 out]
                n988 = property on="ScaleRange" class="Bool (strict)"(error in=w1412, "Val(Sgnl)"=TRUE ("Value (Signaling)")) -> ()  [unwired: 1 in, 2 out]
              }
            }
          }
          frame Enabled {
          }
        }
      }
      event "Scrollbar": Value Change {
        n989 = event-data() -> ("NewVal"=w1417:dbl)  [unwired: 6 out]
        n990 = disable-structure shown="Disabled" {
          disable-tunnel: w1417 -> [w1433 _]
          frame Disabled {
            n991 = local read "ScaleMax"() -> (w1443:dbl)
            n992 = local read "ScaleMin"() -> (w1444:dbl)
            n993 = property on="Scrollbar" class="Scroll (strict)"() -> ("DocMin"=w1442:dbl, "DocMax"=w1441:dbl)  [unwired: 2 in, 2 out]
            n994 = property on="PreviewGraph" class="XYGraph (strict)"("Active Cursor"=u32 0, "Active Cursor"=u32 1) -> ("Cursor.Cursor X"=w1436:dbl, "Cursor.Cursor X"=w1437:dbl)  [unwired: 2 in, 2 out]
            n995 = property on="PreviewGraph" class="XYGraph (strict)"("ActXScl"=0 ("Active X Scale"), "XScale.ScaleFit"=u8 0 ("X Scale.Scale Fit")) -> (error out=w1418:errorcluster)  [unwired: 2 in, 1 out]
            n996 = property on="PreviewGraph" class="XYGraph (strict)"(error in=w1418, "ActXScl"=0 ("Active X Scale")) -> ("XScale.Maximum"=w1429:dbl, "XScale.Minimum"=w1424:dbl)  [unwired: 1 in, 2 out]
            n997 = Subtract(x=w1441, y=w1442) -> (x-y=w1448:dbl)
            n998 = Subtract(x=w1443, y=w1444) -> (x-y=w1446:dbl)
            n999 = Subtract(x=w1433, y=w1442) -> (x-y=w1445:dbl)
            n1000 = Subtract(x=w1436, y=w1437) -> (x-y=w1438:dbl)
            n1001 = Multiply(x=w1445, y=w1446) -> (x*y=w1447:dbl)
            n1002 = Subtract(x=w1429, y=w1424) -> (x-y=w1422:dbl)
            n1003 = Absolute Value(x=w1438) -> (abs(x)=w1423:dbl)
            n1004 = Divide(x=w1447, y=w1448) -> (x/y=w1428:dbl)
            n1005 = Divide(x=w1423, y=w1422) -> (x/y=w1421:dbl)
            n1006 = Less Or Equal To 0?(x=w1438) -> (x <= 0?=w1439:bool)
            n1007 = Add(x=w1421, y=w1428) -> (x+y=w1427:dbl)
            n1008 = Multiply(x=w1422, y=w1428) -> (x*y=w1425:dbl)
            n1009 = Multiply(x=w1422, y=w1427) -> (x*y=w1426:dbl)
            n1010 = Add(x=w1424, y=w1426) -> (x+y=w1431:dbl)
            n1011 = Add(x=w1424, y=w1425) -> (x+y=w1430:dbl)
            n1012 = case shown="True" w1439 {
              tunnel: w1430 -> [w1452 w1457]
              tunnel: w1431 -> [w1451 w1456]
              tunnel: [w1453 w1458] -> w1440
              tunnel: [w1452 w1457] -> w1449
              tunnel: [w1451 w1456] -> w1450
              frame True {
                n1013 = property on="PreviewGraph" class="XYGraph (strict)"("Active Cursor"=u32 0, "Cursor.Cursor X"=w1452, "Active Cursor"=u32 1, "Cursor.Cursor X"=w1451) -> (error out=w1453:errorcluster)  [unwired: 2 in, 1 out]
              }
              frame False {
                n1014 = property on="PreviewGraph" class="XYGraph (strict)"("Active Cursor"=u32 1, "Cursor.Cursor X"=w1457, "Active Cursor"=u32 0, "Cursor.Cursor X"=w1456) -> (error out=w1458:errorcluster)  [unwired: 2 in, 1 out]
              }
            }
            n1015 = property on="XY Graph" class="XYGraph (strict)"("XScale.Minimum"=w1449, "XScale.Maximum"=w1450) -> ()  [unwired: 2 in, 2 out]
            n1016 = flat-sequence {
              tunnel: w1440 -> [_]
              frame #0 {
                n1017 = control-ref of="This VI"() -> (w1462:refnum<vi>)
                n1018 = call "CRYPlot XY Graph Preview.vi"("sOption"="Move", "Graph VI Ref"=w1462) -> ()  [unwired: 10 in]
              }
            }
          }
          frame Enabled {
          }
        }
      }
      event "OpenProperty": Value Change {
        n1019 = event-data() -> ()  [unwired: 7 out]
        n1020 = flat-sequence {
          frame #0 {
            n1021 = local read "PropertyTab"() -> (w1463:string)
            n1022 = control-ref of="This VI"() -> (w1464:refnum<vi>)
            n1023 = call "CRYGraph Property Window Main.vi"("TabName"=w1463, "pGraph VI In"=w1464) -> ()  [unwired: 1 in, 9 out]
          }
          frame #1 {
            n1024 = local write "PropertyTab"("" ("PropertyTab")) -> ()
          }
        }
      }
      event "ToolbarUpdate": Value Change {
        n1025 = event-data() -> ()  [unwired: 7 out]
        n1026 = local read "Test"() -> (w1466:string)
        n1027 = case shown="Default" w1466 {
          frame "Test" {
          }
          frame Default {
            n1028 = local read "Event Name"() -> (w1467:string)
            n1029 = case shown="Default" w1467 {
              frame "ViewReport" {
              }
              frame Default {
                n1030 = control-ref of="This VI"() -> (w1469:refnum<vi>)
                n1031 = call "CRYUpdate DataView Toolbar.vi"("pVI"=w1469) -> ()  [unwired: 11 in]
                n1032 = call "CRYPreUpdate Sequence.vi"("EventName"="CurLibUpdate") -> ()  [unwired: 15 in]
              }
            }
          }
        }
      }
    }
    n1033 = global read "CRYMain Sub Window Global.vi" "gStop"() -> (w126:bool)
    n1034 = Or(x=w126, y="stop") -> (x .or. y?=w122:bool)
  }
  n1035 = while {
    tunnel: w1 -> [w1477]
    shift-right: [w1472] -> w9
    shift-left: w10 -> [w1475]
    stop <- w1478 stop-if-true
    n1036 = Get Queue Status(queue=w1477, error in (no error)=w1475) -> (queue out=w1476:refnum<queue>, error out=w1472:errorcluster, # elements in queue=w1473:i32)  [unwired: 6 out]
    n1037 = Wait (ms)(milliseconds to wait=u32 10) -> ()  [unwired: 1 out]
    n1038 = case shown="Default" w1473 {
      tunnel: w1476 -> [_ w1483]
      tunnel: w1472 -> [_ w1482]
      frame 0 {
        n1039 = Wait (ms)(milliseconds to wait=u32 10) -> ()  [unwired: 1 out]
      }
      frame Default {
        n1040 = Dequeue Element(queue=w1483, error in (no error)=w1482) -> (element=w1480:string, error out=w1481:errorcluster)  [unwired: 3 out]
        n1041 = case shown="No Error" w1481 {
          tunnel: w1480 -> [w1487 _]
          frame No Error {
            n1042 = Scan From String(format string="%s%s%d%d", input string=w1487) -> (output 1=w1485:string, output 2=w1484:string, output 3=w1486:i32)  [unwired: 2 in, 8 out]
            n1043 = case shown="\"Cursor_Move\"" w1485 {
              tunnel: w1486 -> [_ w1494]
              tunnel: w1484 -> [_ w1492]
              frame Default {
              }
              frame "Cursor_Move" {
                n1044 = local read "CursorMoveFinish"() -> (w1490:bool)
                n1045 = local read "WhichKey"() -> (w1493:string)
                n1046 = Equal?(x=w1492, y=w1493) -> (x = y?=w1491:bool)
                n1047 = And(x=w1491, y=w1490) -> (x .and. y?=w1489:bool)
                n1048 = case shown="True" w1489 {
                  tunnel: w1494 -> [_ w1495]
                  frame False {
                  }
                  frame True {
                    n1049 = flat-sequence {
                      tunnel: w1495 -> [w1498]
                      frame #0 {
                        n1050 = local read "NewCursIdx"() -> (w1496:u32)
                        n1051 = control-ref of="XY Graph"() -> (w1497:refnum<vi>)
                        n1052 = call "CRYCursor Move.vi"("x"=w1498, "Active Cursor"=w1496, "Graph Ref"=w1497) -> ()  [unwired: 9 in]
                      }
                      frame #1 {
                        n1053 = local read "CursorShow"() -> (w1499:bool)
                        n1054 = case shown="True" w1499 {
                          frame False {
                          }
                          frame True {
                            n1055 = control-ref of="XY Graph"() -> (w1502:refnum<vi>)
                            n1056 = control-ref of="Cursor"() -> (w1501:refnum<vi>)
                            n1057 = call "CRYPlot Cursor.vi"("Cursor Ref"=w1501, "Graph Ref"=w1502, "Graph Type"="XY") -> ()  [unwired: 9 in]
                          }
                        }
                      }
                    }
                  }
                }
              }
            }
          }
          frame Error {
          }
        }
      }
    }
    n1058 = Unbundle By Name(w1472) -> ("status"=w1471:bool)
    n1059 = local read "stop"() -> (w1470:bool)
    n1060 = Or(x=w1470, y=w1471) -> (x .or. y?=w1478:bool)
  }
  n1061 = Release Queue(queue=w1, error in (no error)=w9) -> (error out=w2:errorcluster)  [unwired: 3 out]
  n1062 = flat-sequence {
    tunnel: w11 -> [_]
    tunnel: w2 -> [_]
    frame #0 {
      n1063 = local write "StateOut"(TRUE ("StateOut")) -> ()
    }
  }
